vi "Main.vi"() -> ()   [LabVIEW 2020]
doc: "This template is for the Queued Message Handler design pattern.\n\nThe Event Handling Loop generates messages based on user interface actions.\n\nThe Message Handling Loop processes messages generated by the Event Handling Loop, or by other messages. The messages are string values, so new messages can be added easily to the Message Cases case structure in the Message Handling Loop. Each message cluster can also provide an optional value for Message Data, which is a variant that can be converted to whatever message-specific data is required."
uses:
  SubVi/TypeDef2ndLoop.ctl
  controls/UI Data.ctl
  <vilib>/Utility/miscctls.llb/LVForegroundBackgroundColorsTypeDef.ctl
  <vilib>/Utility/miscctls.llb/LVStringsAndValuesArrayTypeDef_U16.ctl
  <vilib>/Analysis/3filter.llb/Savitzky-Golay Filter (DBL).vi
  support/Message Queue/Enqueue Message (Single).vi
  <vilib>/Utility/file.llb/Write Delimited Spreadsheet (DBL).vi
  <vilib>/Utility/error.llb/Error Cluster From Error Code.vi
  <vilib>/ErrorRing/Error Ring.xnode
  <vilib>/Analysis/6fits.llb/Confidence Interval (Gauss).vi
  support/Message Queue/Message Queue.lvlib
  support/User Event - Stop/User Event - Stop.lvlib
  <instrlib>/Ocean Optics 2000 4000/Ocean Optics 2000 4000.lvlib
  <vilib>/Analysis/NI_AALBase.lvlib
  <vilib>/Analysis/NI_AALPro.lvlib
panel:
  out "PlotMouseFollow":string
  in  "Tab Control":enum32{"Analysis and Aquisition", "HR4000 "}(tab)
  in  "Grid on graph":bool
  in  "20(I)/10(P)":bool
  in  "Intensity/dB":bool
  in  "AutoScale":bool
  in  "Tab small":enum32{"Data Operations", "Linfit View"}(tab)
  in  "Save to file 3":bool
  in  "FIlterType":u16(ring) items=["Savitzky-Golay"]
  in  "FIlterorder":u16(ring) items=["1st order poly.", "2nd order poly.", "3rd order poly.", "4th order poly.", "5th order poly. ", "6th order poly."]
  in  "Filter":bool
  in  "Remove negative values":bool
  out "Data(X/Y)":cluster{dbl[], dbl[]}[](array[cluster])
  in  "Interpolate":bool
  in  "PlotChooser 2":u16(ring) items=["6,5cm60000"]
  in  "MathNumber":dbl
  in  "Math":bool
  in  "Tab Math":u16(ring) items=["Multiply", "Divide", "Add", "Decrement"]
  in  "Normalise":bool
  in  "Save to file":bool
  out "Max":dbl
  out "Min":dbl
  out "Attenuation[dB/cm]":dbl
  out "Linfit":cluster{"X":dbl[], "Best Linear Fit":dbl[]}[](graph)
  out "Intercept":dbl
  in  "Save session":bool
  out "FWHM":dbl
  in  "End":dbl min=0.0 max=2000.0
  in  "Start":dbl min=0.0 max=2000.0
  out "Attenuation[dB/cm]":dbl
  in  "Reference":dbl
  out "Reference name":string
  out "Attenuation[dB]":string
  out "Integral":string
  in  "PlotChooser":u16(ring) items=["6,5cm60000"]
  in  "DownloadData":bool
  out "Spectras-Analiza":cluster{dbl[], dbl[]}[](graph)
  in  "Delete series":bool
  in  "Data Display":dbl[][](array[numeric])
  out "Lenght[cm]":string
  in  "LinearFit":bool
  in  "Light mode":bool
  in  "Grid":bool
  in  "Intensity/dB":bool
  in  "Delete last":bool
  in  "PlotChooser 3":u16(ring) items=["Aquired"]
  in  "DarkSpectrum":bool
  in  "Save current spectrum":bool
  out "Spectras-Analiza 2":cluster{dbl[], dbl[]}[](graph)
  in  "VISA resource name":refnum<visa-resource-name>
  in  "Connect":bool
  in  "Disconnect":bool
  in  "Integration time [us]":i32=1 min=1 max=500000
  in  "Send data":bool
  out "Connection status":errorcluster
  in  "Choose folder":path
  in  "Save to file 2":bool
  in  "Aquire":bool
  in  "AutoScale":bool
  in  "AqvOverTime":bool
  in  "Exit":bool
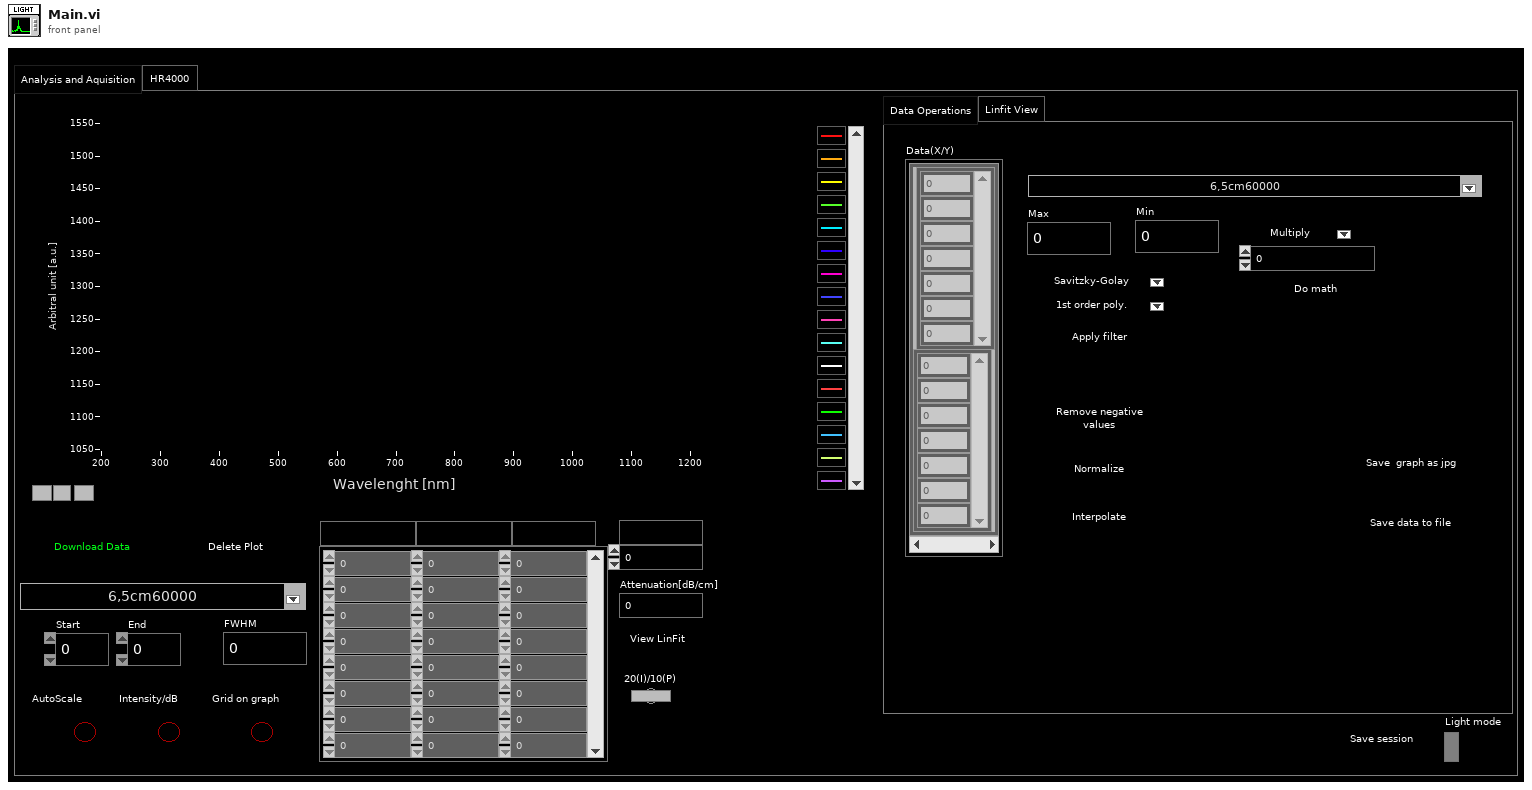
[diagram p1: front panel]
types:
  T1 = typedef "UI Data.ctl" = cluster{"Exit Button Ref":refnum<vi>, "Spectras-Analiza":cluster{dbl[], dbl[]}[], "PlotNumber":dbl, "DataDisplay":dbl[][], "VISA resource name":refnum<visa-resource-name>, "VISA error cluster":errorcluster, "Names of plots":cluster{"Plot.Plot Name":string, i32}[]}
  T2 = typedef "TypeDef2ndLoop.ctl" = cluster{"VISA resource name":refnum<visa-resource-name>, "VISA error cluster":errorcluster, "Spectras-Analiza":cluster{dbl[], dbl[]}[], "Spectral Waveform":cluster{dbl[], dbl[]}, "Spectrum by Pixel Number":dbl[], "Dark?":bool}
  T3 = typedef "Message Queue.lvlib/All Message Queues.ctl" = cluster{"1stloop":refnum<queue>, "2ndLoop":refnum<queue>}
  T4 = typedef "LVStringsAndValuesArrayTypeDef_U16.ctl" = cluster{"String":string, "Value":u16}[]
  T5 = enum8{"Enabled", "Disabled", "Disabled and Grayed Out"}
  T6 = cluster{"Wavelength (nm)":dbl[], "Spectrum by Pixel Number":dbl[]}
  T7 = typedef "LVForegroundBackgroundColorsTypeDef.ctl" = cluster{"Foreground Color":u32, "Background Color":u32}
  T8 = cluster{"name (change?)":string, "PlotNumber":dbl}[]
  T9 = typedef "LVPoint32TypeDef.ctl" = cluster{"Horizontal":i32, "Vertical":i32}
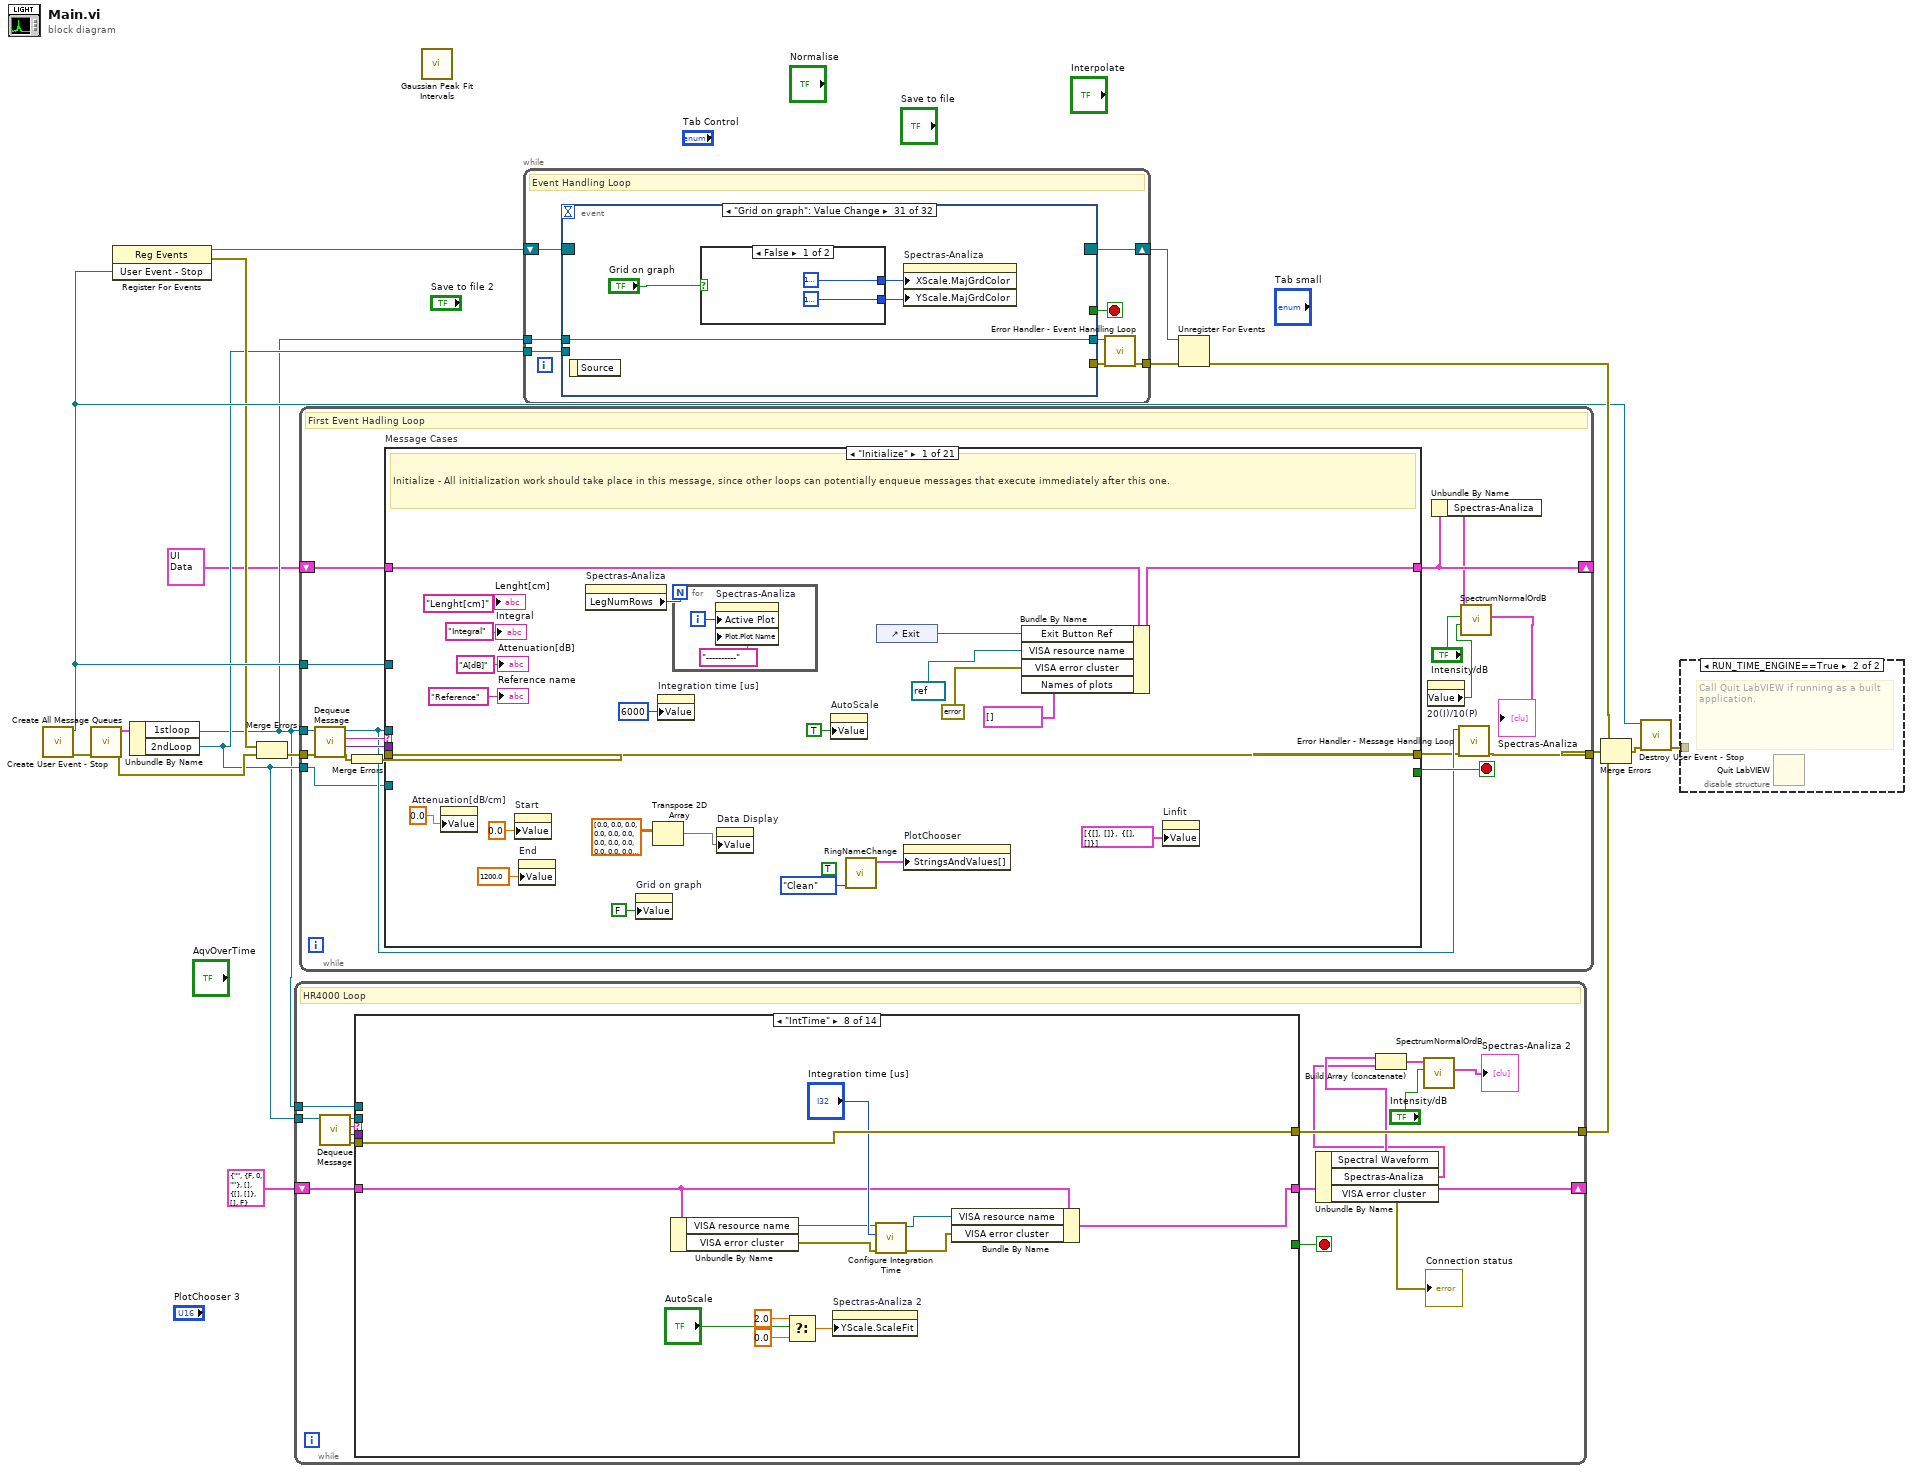
[diagram p0: block diagram]
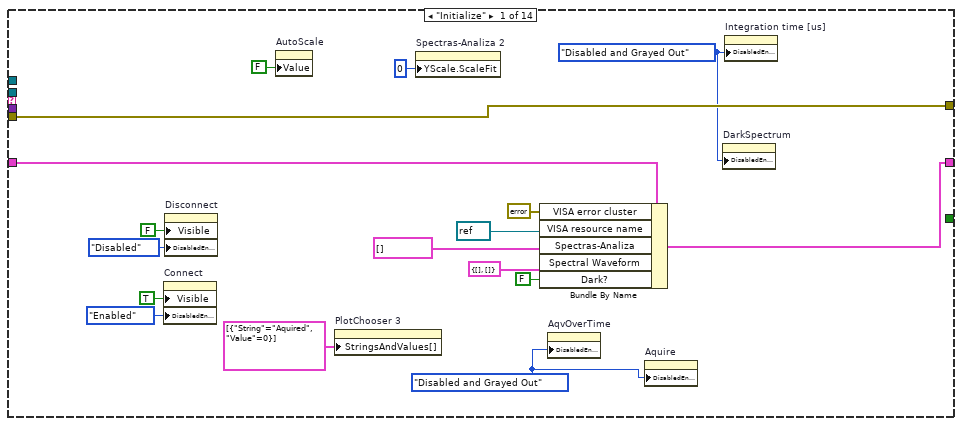
[diagram p2: hidden frame]
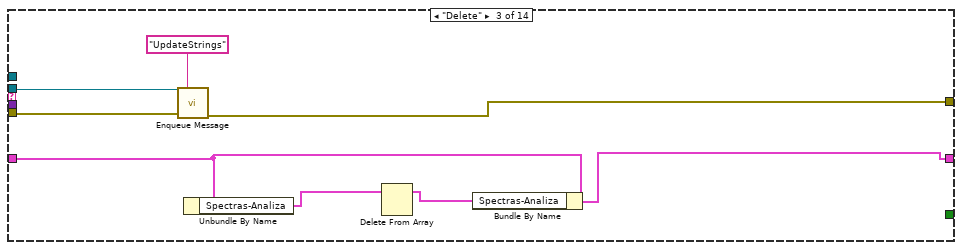
[diagram p4: hidden frame]
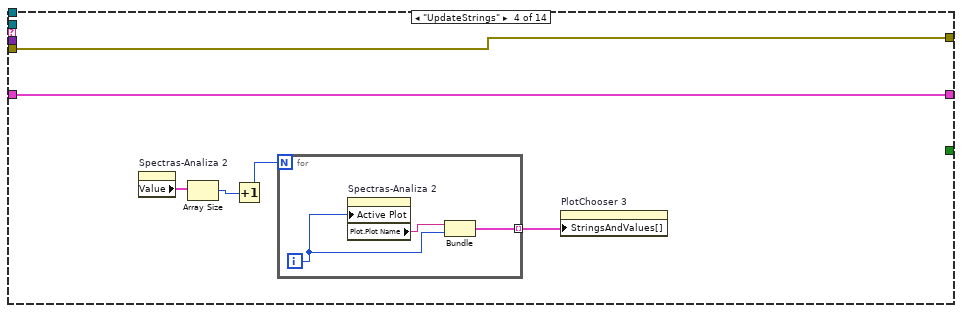
[diagram p5: hidden frame]
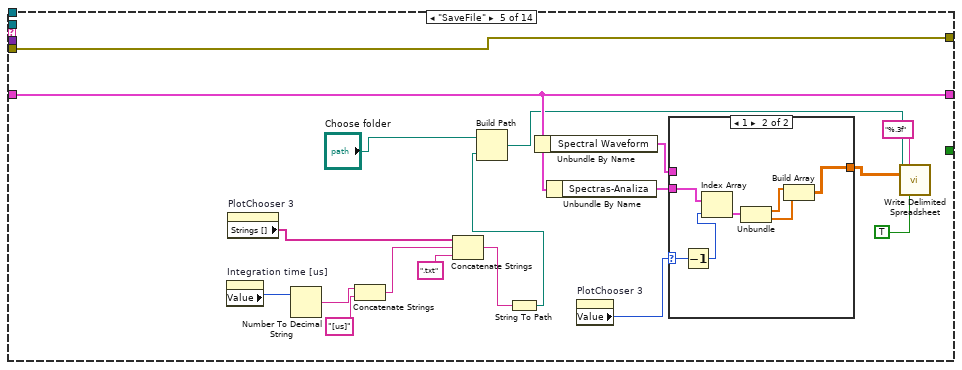
[diagram p6: hidden frame]
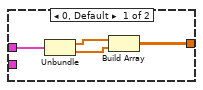
[diagram p7: hidden frame]
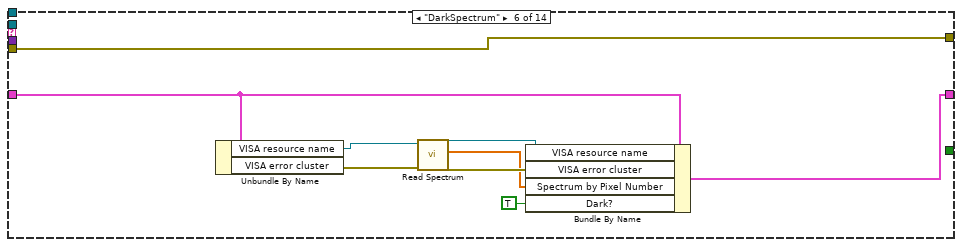
[diagram p8: hidden frame]
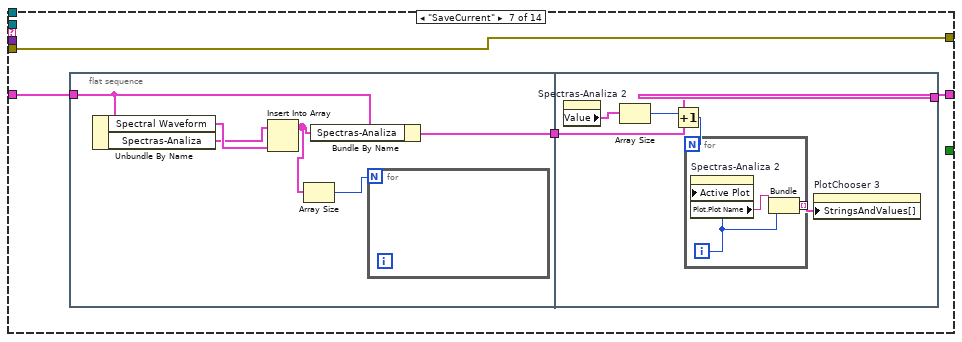
[diagram p9: hidden frame]
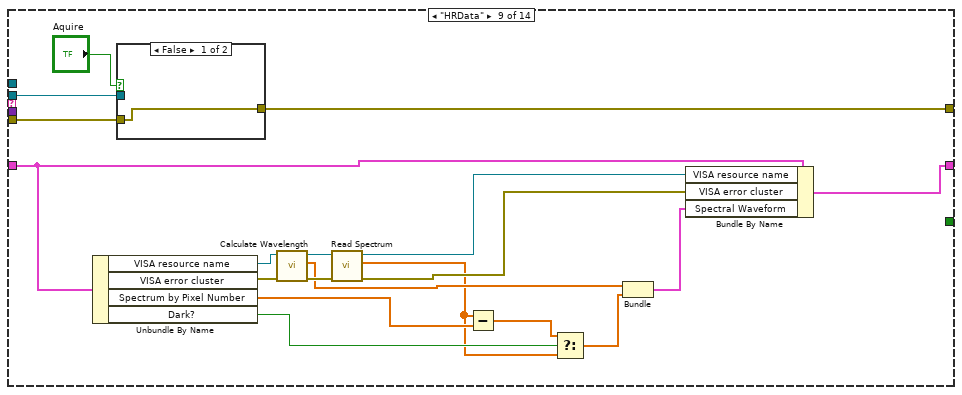
[diagram p10: hidden frame]
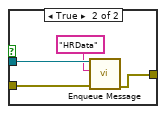
[diagram p11: hidden frame]
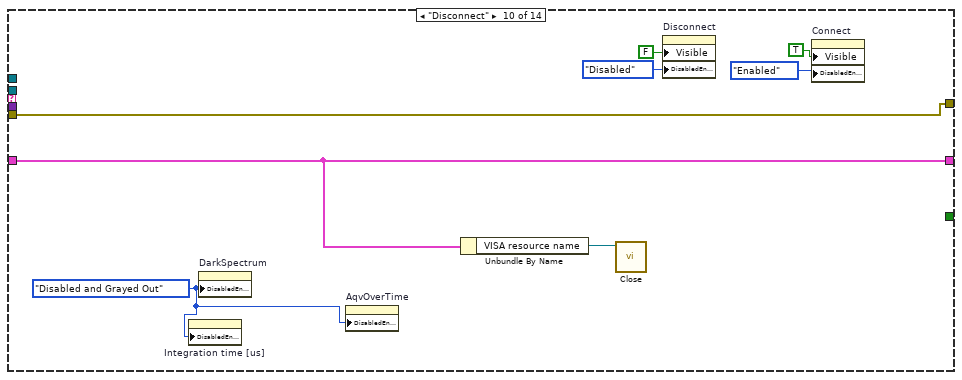
[diagram p12: hidden frame]
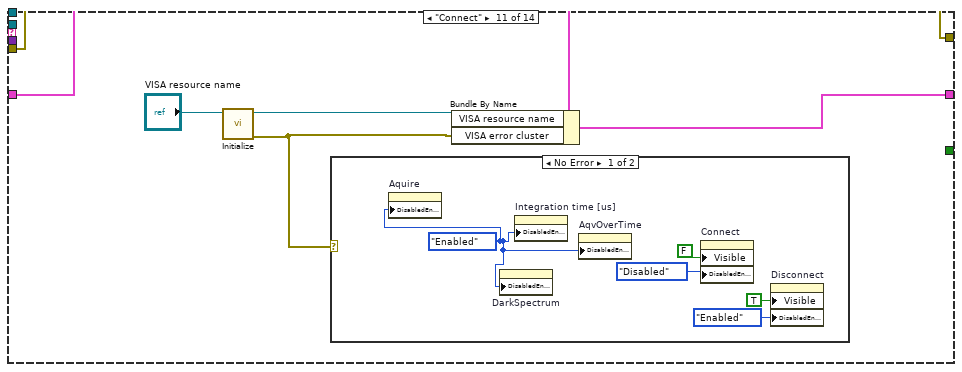
[diagram p13: hidden frame]
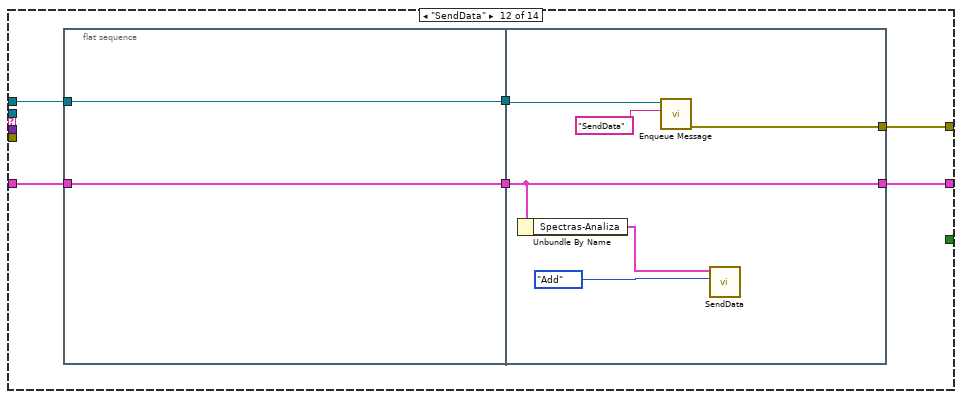
[diagram p15: hidden frame]
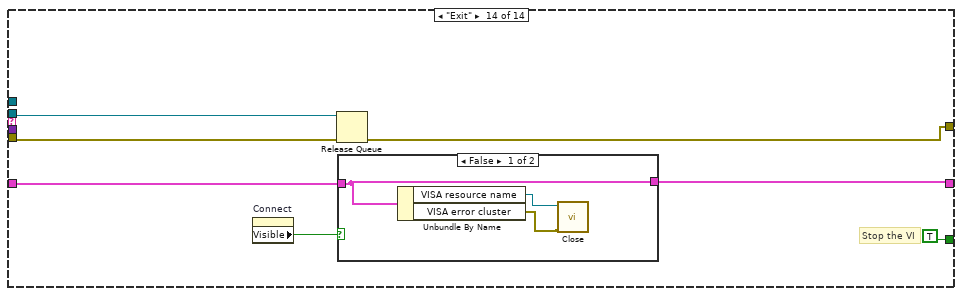
[diagram p17: hidden frame]
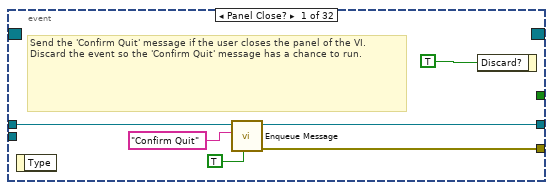
[diagram p20: hidden frame]
diagram:
  n1 = call "Create User Event - Stop.vi"() -> ("error out"=w15:errorcluster, "User Event - Stop"=w8:refnum<user-event>)  [unwired: 10 in]
  n2 = call "Create All Message Queues.vi"("error in (no error)"=w15) -> ("error out"=w18:errorcluster, "Message Queues out"=w17:T3)  [unwired: 9 in]
  n3 = register-events(w8) -> (reference out=w9:refnum<event-registration>, error out=w6:errorcluster)  [unwired: 2 in]
  n4 = Unbundle By Name(w17) -> ("1stloop"=w3:refnum<queue>, "2ndLoop"=w4:refnum<queue>)
  n5 = Merge Errors(w6, w18) -> (w7:errorcluster)
  n6 = while {
    tunnel: w4 -> [w33]
    tunnel: [w28] -> w5
    tunnel: w3 -> [w27]
    shift-right: [w25] -> _
    shift-left: T2 {"VISA resource name"="", "VISA error cluster"={"status"=FALSE, "code"=0, "source"=""}, "Spectras-Analiza"=[], "Spectral Waveform"={[], []}, "Spectrum by Pixel Number"=[], "Dark?"=FALSE} -> [w26]
    stop <- w34 stop-if-true
    # "HR4000 Loop"
    n7 = call "Dequeue Message.vi"("Message Queue"=w33) -> ("error out"=w30:errorcluster, "Message Data"=w31:variant, "Message"=w32:string, "dup Message Queue"=w29:refnum<queue>)  [unwired: 7 in]
    n8 = case shown="\"IntTime\"" w32 {
      tunnel: [_ _ _ _ _ _ _ _ _ _ _ _ _ TRUE] -> w34
      tunnel: w31 -> [_ _ _ _ _ _ _ _ _ _ _ _ _ _]
      tunnel: w30 -> [w51 w53 w56 w67 w88 w108 w112 w138 w155 w164 w172 _ w197 w202]
      tunnel: w29 -> [_ _ w57 _ _ _ _ _ w153 _ _ _ _ w203]
      tunnel: [w51 w53 w55 w67 w88 w108 w112 w138 w154 w164 w172 w185 w197 w198] -> w28
      tunnel: w27 -> [_ _ _ _ _ _ _ _ _ _ _ w187 _ _]
      tunnel: w26 -> [w49 w52 w60 w66 w77 w105 w111 w134 w157 w165 w176 w182 w196 w200]
      tunnel: [w50 w52 w58 w66 w77 w101 w110 w131 w156 w165 w175 w184 w196 w199] -> w25
      frame "Initialize" {
        w35 = T5."Disabled and Grayed Out" ("Disabled")
        w37 = T5."Disabled and Grayed Out" ("Disabled")
        n9 = property on="Connect" class="Bool"("Visible"=TRUE, "DisabledEnum"=T5."Enabled" ("Disabled")) -> ()  [unwired: 2 in, 2 out]
        n10 = property on="Disconnect" class="Bool"("Visible"=FALSE, "DisabledEnum"=T5."Disabled" ("Disabled")) -> ()  [unwired: 2 in, 2 out]
        n11 = property on="AutoScale" class="Bool (strict)"("Value"=FALSE ("AutoScale")) -> ()  [unwired: 2 in, 2 out]
        n12 = property on="PlotChooser 3" class="Ring (strict)"("StringsAndValues[]"=T4 [{"String"="Aquired", "Value"=0}] ("Strings And Values []")) -> ()  [unwired: 2 in, 2 out]
        n13 = property on="Spectras-Analiza 2" class="XYGraph (strict)"("YScale.ScaleFit"=u8 0 ("Y Scale.Scale Fit")) -> ()  [unwired: 2 in, 2 out]
        n14 = Bundle By Name(cluster=w49, "VISA error cluster"=errorcluster {"status"=FALSE, "code"=0, "source"=""}, "VISA resource name"=refnum<visa-resource-name> refnum, "Spectras-Analiza"=cluster{dbl[], dbl[]}[] [], "Spectral Waveform"=cluster{dbl[], dbl[]} {[], []}, "Dark?"=FALSE) -> (w50:T2)
        n15 = property on="AqvOverTime" class="Bool (strict)"("DisabledEnum"=w35) -> ()  [unwired: 2 in, 2 out]
        n16 = property on="Aquire" class="Bool (strict)"("DisabledEnum"=w35) -> ()  [unwired: 2 in, 2 out]
        n17 = property on="DarkSpectrum" class="Bool"("DisabledEnum"=w37) -> ()  [unwired: 2 in, 2 out]
        n18 = property on="Integration time [us]" class="DigNum (strict)"("DisabledEnum"=w37) -> ()  [unwired: 2 in, 2 out]
      }
      frame "---Copy This Case---" {
      }
      frame "Delete" {
        n19 = call-poly "Enqueue Message.vi"("error in (no error)"=w56, "Message"="UpdateStrings", "Message Queue"=w57) -> ("error out"=w55:errorcluster)  [unwired: 7 in, 1 out]
        n20 = Unbundle By Name(w60) -> ("Spectras-Analiza"=w61:cluster{dbl[], dbl[]}[])
        n21 = Delete From Array(array=w61) -> (array with subset deleted=w59:cluster{dbl[], dbl[]}[])  [unwired: 2 in, 1 out]
        n22 = Bundle By Name(cluster=w60, "Spectras-Analiza"=w59) -> (w58:T2)
      }
      frame "UpdateStrings" {
        n23 = property on="Spectras-Analiza 2" class="XYGraph (strict)"() -> ("Value"=w65:cluster{dbl[], dbl[]}[])  [unwired: 2 in, 2 out]
        n24 = Array Size(array=w65) -> (size(s)=w64:i32)
        n25 = Increment(x=w64) -> (x+1=w63:i32)
        n26 = for {
          N: w63 -> [_]
          tunnel: [w68] -> w62 mode=indexing
          i -> [w69]
          n27 = property on="Spectras-Analiza 2" class="XYGraph (strict)"("Active Plot"=w69) -> ("Plot.Plot Name"=w70:string)  [unwired: 2 in, 2 out]
          n28 = Bundle("Plot.Plot Name"=w70, w69) -> (w68:cluster{"Plot.Plot Name":string, i32})  [unwired: 1 in]
        }
        n29 = property on="PlotChooser 3" class="Ring (strict)"("StringsAndValues[]"=w62) -> ()  [unwired: 2 in, 2 out]
      }
      frame "SaveFile" {
        n30 = property on="Integration time [us]" class="DigNum (strict)"() -> ("Value"=w83:i32)  [unwired: 2 in, 2 out]
        n31 = property on="PlotChooser 3" class="Ring (strict)"() -> ("Strings []"=w85:string[])  [unwired: 2 in, 2 out]
        n32 = Number To Decimal String(number=w83) -> (decimal integer string=w82:string)  [unwired: 1 in]
        n33 = Concatenate Strings(w82, "[us]" ("string")) -> (w80:string)
        n34 = Concatenate Strings(w85, w80, ".txt" ("string")) -> (w86:string)
        n35 = String To Path(string=w86) -> (path=w79:path)
        n36 = Build Path(base path="Choose folder", name or relative path=w79) -> (appended path=w74:path)
        n37 = Unbundle By Name(w77) -> ("Spectral Waveform"=w76:cluster{dbl[], dbl[]})
        n38 = Unbundle By Name(w77) -> ("Spectras-Analiza"=w75:cluster{dbl[], dbl[]}[])
        n39 = property on="PlotChooser 3" class="Ring (strict)"() -> ("Value"=w78:u16)  [unwired: 2 in, 2 out]
        n40 = case shown="1" w78 {
          selector: w78 -> [_ w98]
          tunnel: w76 -> [w92 _]
          tunnel: [w89 w93] -> w71
          tunnel: w75 -> [_ w99]
          frame 0, Default {
            n41 = Unbundle(w92) -> (w91:dbl[], w90:dbl[])
            n42 = Build Array(w91, w90) -> (w89:dbl[][])
          }
          frame 1 {
            n43 = Decrement(x=w98) -> (x-1=w97:u16)
            n44 = Index Array(array=w99, index=w97) -> (element=w96:cluster{dbl[], dbl[]})
            n45 = Unbundle(w96) -> (w95:dbl[], w94:dbl[])
            n46 = Build Array(w95, w94) -> (w93:dbl[][])
          }
        }
        n47 = call-poly <vilib>:"Write Delimited Spreadsheet.vi"("file path (dialog if empty)"=w74, "format (%.3f)"="%.3f", "2D data"=w71, "transpose? (no:F)"=TRUE) -> ()  [unwired: 10 in, 2 out]
      }
      frame "DarkSpectrum" {
        n48 = Unbundle By Name(w105) -> ("VISA resource name"=w107:refnum<visa-resource-name>, "VISA error cluster"=w106:errorcluster)
        n49 = call <instrlib>:"Read Spectrum.vi"("error in (no error)"=w106, "VISA resource name"=w107) -> ("error out"=w103:errorcluster, "Spectrum by Pixel Number"=w102:dbl[], "VISA resource name out"=w104:refnum<visa-resource-name>)  [unwired: 6 in, 1 out]
        n50 = Bundle By Name(cluster=w105, "VISA resource name"=w104, "VISA error cluster"=w103, "Spectrum by Pixel Number"=w102, "Dark?"=TRUE) -> (w101:T2)
      }
      frame "SaveCurrent" {
        n51 = flat-sequence {
          tunnel: w111 -> [w116]
          tunnel: [w115] -> w109
          tunnel: [w123] -> w110
          tunnel: w109 -> [w123]
          frame #0 {
            n52 = Unbundle By Name(w116) -> ("Spectral Waveform"=w118:cluster{dbl[], dbl[]}, "Spectras-Analiza"=w117:cluster{dbl[], dbl[]}[])
            n53 = Insert Into Array(array=w117, new element=w118) -> (w114:cluster{dbl[], dbl[]}[])  [unwired: 1 in]
            n54 = Array Size(array=w114) -> (size(s)=w113:i32)
            n55 = Bundle By Name(cluster=w116, "Spectras-Analiza"=w114) -> (w115:T2)
            n56 = for {
              N: w113 -> [_]
            }
          }
          frame #1 {
            n57 = property on="Spectras-Analiza 2" class="XYGraph (strict)"() -> ("Value"=w122:cluster{dbl[], dbl[]}[])  [unwired: 2 in, 2 out]
            n58 = Array Size(array=w122) -> (size(s)=w121:i32)
            n59 = Increment(x=w121) -> (x+1=w120:i32)
            n60 = for {
              N: w120 -> [_]
              tunnel: [w124] -> w119 mode=indexing
              i -> [w125]
              n61 = property on="Spectras-Analiza 2" class="XYGraph (strict)"("Active Plot"=w125) -> ("Plot.Plot Name"=w126:string)  [unwired: 2 in, 2 out]
              n62 = Bundle("Plot.Plot Name"=w126, w125) -> (w124:cluster{"Plot.Plot Name":string, i32})  [unwired: 1 in]
            }
            n63 = property on="PlotChooser 3" class="Ring (strict)"("StringsAndValues[]"=w119) -> ()  [unwired: 2 in, 2 out]
          }
        }
      }
      frame "IntTime" {
        n64 = Unbundle By Name(w134) -> ("VISA resource name"=w136:refnum<visa-resource-name>, "VISA error cluster"=w135:errorcluster)
        n65 = Select(t=2.0, s="AutoScale", f=0.0) -> (s? t:f=w129:dbl)
        n66 = property on="Spectras-Analiza 2" class="XYGraph (strict)"("YScale.ScaleFit"=w129) -> ()  [unwired: 2 in, 2 out]
        n67 = call <instrlib>:"Configure Integration Time.vi"("error in (no error)"=w135, "Integration Time (6000)"="Integration time [us]", "VISA resource name"=w136) -> ("error out"=w132:errorcluster, "VISA resource name out"=w133:refnum<visa-resource-name>)  [unwired: 7 in]
        n68 = Bundle By Name(cluster=w134, "VISA resource name"=w133, "VISA error cluster"=w132) -> (w131:T2)
      }
      frame "HRData" {
        n69 = Unbundle By Name(w157) -> ("VISA resource name"=w150:refnum<visa-resource-name>, "VISA error cluster"=w149:errorcluster, "Spectrum by Pixel Number"=w143:dbl[], "Dark?"=w142:bool)
        n70 = case shown="False" "Aquire" {
          tunnel: w155 -> [w158 w162]
          tunnel: [w158 w161] -> w154
          tunnel: w153 -> [_ w160]
          frame False {
          }
          frame True {
            n71 = call-poly "Enqueue Message.vi"("error in (no error)"=w162, "Message"="HRData", "Message Queue"=w160) -> ("error out"=w161:errorcluster)  [unwired: 7 in, 1 out]
          }
        }
        n72 = call <instrlib>:"Calculate Wavelength.vi"("error in (no error)"=w149, "VISA resource name"=w150) -> ("error out"=w148:errorcluster, "Wavelength (nm)"=w145:dbl[], "VISA resource name out"=w151:refnum<visa-resource-name>)  [unwired: 1 in, 6 out]
        n73 = call <instrlib>:"Read Spectrum.vi"("error in (no error)"=w148, "VISA resource name"=w151) -> ("error out"=w146:errorcluster, "Spectrum by Pixel Number"=w140:dbl[], "VISA resource name out"=w147:refnum<visa-resource-name>)  [unwired: 6 in, 1 out]
        n74 = Subtract(x=w140, y=w143) -> (x-y=w141:dbl[])
        n75 = Select(t=w141, s=w142, f=w140) -> (s? t:f=w139:dbl[])
        n76 = Bundle("Wavelength (nm)"=w145, "Spectrum by Pixel Number"=w139) -> (w144:T6)  [unwired: 1 in]
        n77 = Bundle By Name(cluster=w157, "VISA resource name"=w147, "VISA error cluster"=w146, "Spectral Waveform"=w144) -> (w156:T2)
      }
      frame "Disconnect" {
        w163 = T5."Disabled and Grayed Out" ("Disabled")
        n78 = property on="Integration time [us]" class="DigNum (strict)"("DisabledEnum"=w163) -> ()  [unwired: 2 in, 2 out]
        n79 = property on="DarkSpectrum" class="Bool"("DisabledEnum"=w163) -> ()  [unwired: 2 in, 2 out]
        n80 = property on="AqvOverTime" class="Bool (strict)"("DisabledEnum"=w163) -> ()  [unwired: 2 in, 2 out]
        n81 = Unbundle By Name(w165) -> ("VISA resource name"=w170:refnum<visa-resource-name>)
        n82 = call <instrlib>:"Close.vi"("VISA resource name"=w170) -> ()  [unwired: 10 in, 1 out]
        n83 = property on="Disconnect" class="Bool"("Visible"=FALSE, "DisabledEnum"=T5."Disabled" ("Disabled")) -> ()  [unwired: 2 in, 2 out]
        n84 = property on="Connect" class="Bool"("Visible"=TRUE, "DisabledEnum"=T5."Enabled" ("Disabled")) -> ()  [unwired: 2 in, 2 out]
      }
      frame "Connect" {
        n85 = call <instrlib>:"Initialize.vi"("VISA resource name"="VISA resource name") -> ("error out"=w171:errorcluster, "VISA resource name out"=w173:refnum<visa-resource-name>)  [unwired: 9 in]
        n86 = case shown="No Error" w171 {
          frame No Error {
            w177 = T5."Enabled" ("Disabled")
            n87 = property on="Aquire" class="Bool (strict)"("DisabledEnum"=w177) -> ()  [unwired: 2 in, 2 out]
            n88 = property on="DarkSpectrum" class="Bool"("DisabledEnum"=w177) -> ()  [unwired: 2 in, 2 out]
            n89 = property on="Integration time [us]" class="DigNum (strict)"("DisabledEnum"=w177) -> ()  [unwired: 2 in, 2 out]
            n90 = property on="AqvOverTime" class="Bool (strict)"("DisabledEnum"=w177) -> ()  [unwired: 2 in, 2 out]
            n91 = property on="Connect" class="Bool"("Visible"=FALSE, "DisabledEnum"=T5."Disabled" ("Disabled")) -> ()  [unwired: 2 in, 2 out]
            n92 = property on="Disconnect" class="Bool"("Visible"=TRUE, "DisabledEnum"=T5."Enabled" ("Disabled")) -> ()  [unwired: 2 in, 2 out]
          }
          frame Error {
          }
        }
        n93 = Bundle By Name(cluster=w176, "VISA resource name"=w173, "VISA error cluster"=w171) -> (w175:T2)
      }
      frame "SendData" {
        n94 = flat-sequence {
          tunnel: w187 -> [w189]
          tunnel: [w189] -> w186
          tunnel: [w188] -> w183
          tunnel: w182 -> [w188]
          tunnel: w186 -> [w194]
          tunnel: [w193] -> w185
          tunnel: [w191] -> w184
          tunnel: w183 -> [w191]
          frame #0 {
          }
          frame #1 {
            n95 = Unbundle By Name(w191) -> ("Spectras-Analiza"=w190:cluster{dbl[], dbl[]}[])
            n96 = call-poly "Enqueue Message.vi"("Message"="SendData", "Message Queue"=w194) -> ("error out"=w193:errorcluster)  [unwired: 8 in, 1 out]
            n97 = call "SendData.vi"("Enum"=enum16{"Add", "Take"}."Add", "Spectras-Analiza"=w190) -> ()  [unwired: 9 in, 1 out]
          }
        }
      }
      frame Default {
      }
      frame "Exit" {
        # "Stop the VI"
        n98 = property on="Connect" class="Bool"() -> ("Visible"=w201:bool)  [unwired: 2 in, 2 out]
        n99 = Release Queue(queue=w203, error in (no error)=w202) -> (error out=w198:errorcluster)  [unwired: 1 in, 2 out]
        n100 = case shown="False" w201 {
          tunnel: [w205 w208] -> w199
          tunnel: w200 -> [w205 w208]
          frame False {
            n101 = Unbundle By Name(w205) -> ("VISA resource name"=w207:refnum<visa-resource-name>, "VISA error cluster"=w206:errorcluster)
            n102 = call <instrlib>:"Close.vi"("error in (no error)"=w206, "VISA resource name"=w207) -> ()  [unwired: 9 in, 1 out]
          }
          frame True {
          }
        }
      }
    }
    n103 = Unbundle By Name(w25) -> ("Spectral Waveform"=w24:cluster{dbl[], dbl[]}, "Spectras-Analiza"=w23:cluster{dbl[], dbl[]}[], "VISA error cluster"=→"Connection status":errorcluster)
    n104 = Build Array (concatenate)(w24, w23) -> (w21:cluster{dbl[], dbl[]}[])
    n105 = call "SpectrumNormalOrdB.vi"("Normal/dB"="Intensity/dB", "Spectras-Analiza"=w21) -> ("Spectras-Analiza"=→"Spectras-Analiza 2":cluster{dbl[], dbl[]}[])  [unwired: 9 in]
  }
  n106 = while {
    tunnel: w3 -> [w220]
    shift-right: [w210] -> _
    shift-left: T1 {"Exit Button Ref"=refnum, "Spectras-Analiza"=[], "PlotNumber"=0.0, "DataDisplay"=[[0.0, 0.0, 0.0, 0.0, 0.0, 0.0, 0.0, 0.0, 0.0, 0.0], [0.0, 0.0, 0.0, 0.0, 0.0, 0.0, 0.0, 0.0, 0.0, 0.0], [0.0, 0.0, 0.0, 0.0, 0.0, 0.0, 0.0, 0.0, 0.0, 0.0]], "VISA resource name"="", "VISA error cluster"={"status"=FALSE, "code"=0, "source"=""}, "Names of plots"=[]} ("Data Cluster") -> [w226]
    tunnel: w8 -> [w224]
    tunnel: w7 -> [w223]
    tunnel: [w218] -> w16
    tunnel: w4 -> [w214]
    stop <- w225 stop-if-true
    # "First Event Hadling Loop"
    n107 = call "Dequeue Message.vi"("error in (no error)"=w223, "Message Queue"=w220) -> ("error out"=w216:errorcluster, "Message Data"=w221:variant, "Message"=w222:string, "dup Message Queue"=w219:refnum<queue>)  [unwired: 6 in]
    n108 = Merge Errors(w216) -> (w215:errorcluster)
    n109 = case "Message Cases" shown="\"Initialize\"" w222 {
      selector: w222 -> [_ _ _ _ _ _ _ _ _ _ _ _ _ _ _ _ _ _ _ _ w648]
      tunnel: w219 -> [_ w254 _ w269 w280 w295 w364 w383 _ w405 _ _ w439 w486 w546 w577 w603 _ _ w647 _]
      tunnel: w215 -> [w247 w252 w260 w268 w282 _ w366 w384 w402 w406 w417 w426 w442 w497 w549 w576 w602 w622 w632 w635 _]
      tunnel: [w247 w256 w258 w278 w293 w300 w378 w392 w401 w411 w415 w425 w444 w487 w553 w578 w609 w621 w626 w644 w649] -> w217
      tunnel: w226 -> [w232 w257 w259 w271 w288 w298 w350 w391 w400 w403 w416 w423 w443 w493 w552 w573 w610 w620 w631 w633 w650]
      tunnel: [w249 w257 w259 w270 w283 w299 w343 w391 w400 w410 w416 w423 w438 w490 w551 w574 w610 w620 w631 w633 w650] -> w210
      tunnel: [_ _ _ _ _ _ _ _ _ _ _ _ _ _ _ _ _ _ _ TRUE _] -> w225
      tunnel: w221 -> [_ _ _ _ _ _ _ _ _ _ _ _ _ _ _ _ _ _ w630 w639 _]
      tunnel: w224 -> [_ _ _ _ _ _ _ _ _ _ _ _ _ _ _ _ _ _ _ w643 _]
      tunnel: w214 -> [_ _ _ _ _ _ _ _ _ _ _ _ _ _ _ _ _ _ _ w638 _]
      frame "Initialize" {
        (unwired) TRUE ("Data aquired?")
        # "Initialize - All initialization work should take place in this message, since other loops can potentially enqueue messages that execute immediately after this one."
        n110 = property on="Attenuation[dB/cm]" class="DigNum (strict)"("Value"=0.0 ("Attenuation[all]")) -> ()  [unwired: 2 in, 2 out]
        n111 = property on="Start" class="DigNum (strict)"("Value"=0.0 ("Start")) -> ()  [unwired: 2 in, 2 out]
        n112 = property on="End" class="DigNum (strict)"("Value"=1200.0 ("End")) -> ()  [unwired: 2 in, 2 out]
        n113 = property on="Spectras-Analiza" class="XYGraph (strict)"() -> ("LegNumRows"=w231:u32)  [unwired: 2 in, 2 out]
        n114 = property on="Grid on graph" class="Bool (strict)"("Value"=FALSE ("Grid on graph")) -> ()  [unwired: 2 in, 2 out]
        n115 = Transpose 2D Array(2D array=dbl[][] [[0.0, 0.0, 0.0, 0.0, 0.0, 0.0, 0.0, 0.0, 0.0, 0.0], [0.0, 0.0, 0.0, 0.0, 0.0, 0.0, 0.0, 0.0, 0.0, 0.0], [0.0, 0.0, 0.0, 0.0, 0.0, 0.0, 0.0, 0.0, 0.0, 0.0]] ("Array")) -> (transposed array=w239:dbl[][])
        n116 = property on="Integration time [us]" class="DigNum (strict)"("Value"=6000 ("Integration time")) -> ()  [unwired: 2 in, 2 out]
        n117 = for {
          N: w231 -> [_]
          i -> [w251]
          n118 = property on="Spectras-Analiza" class="XYGraph (strict)"("Active Plot"=w251, "Plot.Plot Name"="----------") -> ()  [unwired: 2 in, 2 out]
        }
        n119 = property on="Data Display" class="Arr (strict)"("Value"=w239) -> ()  [unwired: 2 in, 2 out]
        n120 = property on="AutoScale" class="Bool (strict)"("Value"=TRUE ("AutoScale")) -> ()  [unwired: 2 in, 2 out]
        n121 = call "RingNameChange.vi"("Enum"=enum16{"Add", "Delete", "Clean"}."Clean") -> ("Strings&Arrays"=w237:T8)  [unwired: 10 in]
        n122 = control-ref of="Exit"() -> (w248:refnum<vi>)
        n123 = property on="PlotChooser" class="Ring (strict)"("StringsAndValues[]"=w237) -> ()  [unwired: 2 in, 2 out]
        n124 = Bundle By Name(cluster=w232, "Exit Button Ref"=w248, "VISA resource name"=refnum<visa-resource-name> refnum, "VISA error cluster"=errorcluster {"status"=FALSE, "code"=0, "source"=""}, "Names of plots"=cluster{"Plot.Plot Name":string, i32}[] []) -> (w249:T1)
        n125 = property on="Linfit" class="XYGraph (strict)"("Value"=cluster{"X":dbl[], "Best Linear Fit":dbl[]}[] [{"X"=[], "Best Linear Fit"=[]}, {"X"=[], "Best Linear Fit"=[]}] ("Linfit")) -> ()  [unwired: 2 in, 2 out]
        "Integral" <- "Integral" ("Integral")
        "Lenght[cm]" <- "Lenght[cm]" ("Lenght[cm]")
        "Attenuation[dB]" <- "A[dB]" ("Attenuation[dB]")
        "Reference name" <- "Reference" ("Attenuation[dB] 2")
      }
      frame "Confirm Quit" {
        # "#CodeNeeded - If you want to provide an \"Are you sure\" dialog (or some other notification) before the application exits, place that code here. This message is typically sent from a Panel Close? event."
        # "Confirm Quit - Message that can confirm whether or not the user wants to exit the application."
        n126 = call-poly "Enqueue Message.vi"("error in (no error)"=w252, "Message"="Exit", "Message Queue"=w254) -> ("error out"=w255:errorcluster)  [unwired: 7 in, 1 out]
        n127 = Merge Errors(w255) -> (w256:errorcluster)
      }
      frame "---Copy This Frame---" {
        # "Duplicate this frame when creating new messages.  Change this comment in the duplicated frame to describe this message."
        n128 = Merge Errors(w260) -> (w258:errorcluster)
      }
      frame "Filter" {
        # "Duplicate this frame when creating new messages.  Change this comment in the duplicated frame to describe this message."
        n129 = call-poly "Enqueue Message.vi"("error in (no error)"=w268, "Message"="Integral", "Message Queue"=w269) -> ("error out"=w267:errorcluster)  [unwired: 7 in, 1 out]
        n130 = Unbundle By Name(w271) -> ("Spectras-Analiza"=w264:cluster{dbl[], dbl[]}[])
        n131 = property on="PlotChooser 2" class="Ring (strict)"() -> ("Value"=w272:u16)  [unwired: 2 in, 2 out]
        n132 = Increment(x="FIlterorder") -> (x+1=w261:u16)
        n133 = Index Array(array=w264, index=w272) -> (element=w276:cluster{dbl[], dbl[]})
        n134 = Unbundle(w276) -> (w274:dbl[], w275:dbl[])
        n135 = call-poly <vilib>:"Savitzky-Golay Filter.vi"("polynomial order"=w261, "side points"=6, "X"=w275) -> ("Filtered X"=w273:dbl[])  [unwired: 7 in, 1 out]
        n136 = Bundle(w274, "Filtered X"=w273) -> (w263:cluster{dbl[], "Filtered X":dbl[]})  [unwired: 1 in]
        n137 = Merge Errors(w267) -> (w278:errorcluster)
        n138 = Replace Array Subset(array=w264, new element=w263, index=w272) -> (w262:cluster{dbl[], dbl[]}[])
        n139 = Bundle By Name(cluster=w271, "Spectras-Analiza"=w262) -> (w270:T1)
      }
      frame "DoAbsVal" {
        # "Duplicate this frame when creating new messages.  Change this comment in the duplicated frame to describe this message."
        n140 = call-poly "Enqueue Message.vi"("error in (no error)"=w282, "Message"="Integral", "Message Queue"=w280) -> ("error out"=w281:errorcluster)  [unwired: 7 in, 1 out]
        n141 = Unbundle By Name(w288) -> ("Spectras-Analiza"=w287:cluster{dbl[], dbl[]}[])
        n142 = property on="PlotChooser 2" class="Ring (strict)"() -> ("Value"=w286:u16)  [unwired: 2 in, 2 out]
        n143 = Index Array(array=w287, index=w286) -> (element=w292:cluster{dbl[], dbl[]})
        n144 = Unbundle(w292) -> (w290:dbl[], w291:dbl[])
        n145 = Absolute Value(x=w291) -> (abs(x)=w289:dbl[])
        n146 = Bundle(w290, w289) -> (w285:cluster{dbl[], dbl[]})  [unwired: 1 in]
        n147 = Merge Errors(w281) -> (w293:errorcluster)
        n148 = Replace Array Subset(array=w287, new element=w285, index=w286) -> (w284:cluster{dbl[], dbl[]}[])
        n149 = Bundle By Name(cluster=w288, "Spectras-Analiza"=w284) -> (w283:T1)
      }
      frame "DownloadData" {
        # "Duplicate this frame when creating new messages.  Change this comment in the duplicated frame to describe this message."
        n150 = flat-sequence {
          tunnel: w298 -> [w306]
          tunnel: [w309] -> w297
          tunnel: w295 -> [w301]
          tunnel: [w301] -> w294
          tunnel: [w341] -> w299
          tunnel: w297 -> [w341]
          tunnel: [w339] -> w296
          tunnel: w294 -> [w338]
          frame #0 {
            n151 = call "DownloadDataNewWindow.vi"() -> ("Data aquired?"=w305:bool, "Yaxis"=w307:dbl[], "Xaxis"=w308:dbl[], "name (change?)"=w304:string, "Single FIle?"=w303:bool, "Multiple Data"=w302:cluster{dbl[], dbl[]}[])  [unwired: 6 in]
            n152 = case shown="True" w303 {
              tunnel: [w310 w328] -> w309
              tunnel: w308 -> [_ w325]
              tunnel: w307 -> [_ w324]
              tunnel: w306 -> [w311 w323]
              tunnel: w305 -> [_ w322]
              tunnel: w304 -> [_ w321]
              tunnel: w302 -> [w313 _]
              frame False {
                n153 = Unbundle By Name(w311) -> ("Spectras-Analiza"=w314:cluster{dbl[], dbl[]}[])
                n154 = Insert Into Array(array=w314, new element=w313) -> (w312:cluster{dbl[], dbl[]}[])  [unwired: 1 in]
                n155 = Bundle By Name(cluster=w311, "Spectras-Analiza"=w312) -> (w310:T1)
              }
              frame True {
                n156 = property on="Spectras-Analiza" class="XYGraph (strict)"() -> ("Value"=w318:cluster{dbl[], dbl[]}[])  [unwired: 2 in, 2 out]
                n157 = case shown="True" w322 {
                  tunnel: w321 -> [_ w337]
                  tunnel: w323 -> [w333 w336]
                  tunnel: [w332 w334] -> w320
                  frame False {
                    n158 = Unbundle By Name(w333) -> ("PlotNumber"=w332:dbl)
                  }
                  frame True {
                    n159 = Unbundle By Name(w336) -> ("PlotNumber"=w335:dbl)
                    n160 = property on="Spectras-Analiza" class="XYGraph (strict)"("Active Plot"=w335, "Plot.Plot Name"=w337) -> ()  [unwired: 2 in, 2 out]
                    n161 = Increment(x=w335) -> (x+1=w334:dbl)
                  }
                }
                n162 = Array Size(array=w318) -> (size(s)=w317:i32)
                n163 = Increment(x=w317) -> (x+1=w316:i32)
                n164 = for {
                  N: w316 -> [_]
                  tunnel: [w331] -> w315 mode=indexing
                  i -> [w329]
                  n165 = property on="Spectras-Analiza" class="XYGraph (strict)"("Active Plot"=w329) -> ("Plot.Plot Name"=w330:string)  [unwired: 2 in, 2 out]
                  n166 = Bundle("Plot.Plot Name"=w330, w329) -> (w331:cluster{"Plot.Plot Name":string, i32})  [unwired: 1 in]
                }
                n167 = Unbundle By Name(w323) -> ("Spectras-Analiza"=w327:cluster{dbl[], dbl[]}[])
                n168 = Bundle("Xaxis"=w325, "Yaxis"=w324) -> (w326:cluster{"Xaxis":dbl[], "Yaxis":dbl[]})  [unwired: 1 in]
                n169 = Insert Into Array(array=w327, new element=w326) -> (w319:cluster{dbl[], dbl[]}[])  [unwired: 1 in]
                n170 = property on="PlotChooser" class="Ring (strict)"("StringsAndValues[]"=w315) -> ()  [unwired: 2 in, 2 out]
                n171 = property on="PlotChooser 2" class="Ring (strict)"("StringsAndValues[]"=w315) -> ()  [unwired: 2 in, 2 out]
                n172 = Bundle By Name(cluster=w323, "Spectras-Analiza"=w319, "PlotNumber"=w320, "Names of plots"=w315) -> (w328:T1)
              }
            }
          }
          frame #1 {
            n173 = call-poly "Enqueue Message.vi"("Message"="Integral", "Message Queue"=w338) -> ("error out"=w339:errorcluster)  [unwired: 8 in, 1 out]
          }
        }
        n174 = Merge Errors(w296) -> (w300:errorcluster)
      }
      frame "Integral" {
        # "Duplicate this frame when creating new messages.  Change this comment in the duplicated frame to describe this message."
        n175 = Unbundle By Name(w350) -> ("Spectras-Analiza"=w349:cluster{dbl[], dbl[]}[])
        n176 = property on="PlotChooser 2" class="Ring (strict)"() -> ("Value"=w348:u16)  [unwired: 2 in, 2 out]
        n177 = call-poly "Enqueue Message.vi"("error in (no error)"=w366, "Message"="FWHM", "Message Queue"=w364) -> ("error out"=w365:errorcluster)  [unwired: 7 in, 1 out]
        n178 = property on="20(I)/10(P)" class="Bool (strict)"() -> ("Value"=w351:bool)  [unwired: 2 in, 2 out]
        n179 = Index Array(array=w349, index=w348) -> (element=w347:cluster{dbl[], dbl[]})
        n180 = Unbundle(w347) -> (w346:dbl[])  [unwired: 1 out]
        n181 = call "LinearFit.vi"("End"="End", "Start"="Start", "10/20"=w351, "Data Cluster"=w350) -> ("X"=w359:dbl[], "intercept"=→"Intercept":dbl, "Best Linear Fit"=w360:dbl[], "slope"=→"Attenuation[dB/cm]" →"Attenuation[dB/cm]":dbl, "Y"=w358:dbl[])  [unwired: 3 in]
        n182 = Array Max & Min(array=w346) -> (max value=→"Max":dbl, min value=→"Min":dbl)  [unwired: 2 out]
        n183 = Bundle("X"=w359, "Y"=w358) -> (w357:cluster{"X":dbl[], "Y":dbl[]})  [unwired: 1 in]
        n184 = Bundle("X"=w359, "Best Linear Fit"=w360) -> (w356:cluster{"X":dbl[], "Best Linear Fit":dbl[]})  [unwired: 1 in]
        n185 = Build Array(w357, w356) -> (→"Linfit":cluster{"X":dbl[], "Best Linear Fit":dbl[]}[])
        n186 = property on="20(I)/10(P)" class="Bool (strict)"() -> ("Value"=w352:bool)  [unwired: 2 in, 2 out]
        n187 = Equal?(x="Reference", y=0.0) -> (x = y?=w375:bool)
        n188 = call "DataDisplaySubVi.vi"("End"="End", "Start"="Start", "10/20"=w352, "Reference"="Reference", "Data Display"="Data Display", "Data Cluster"=w350) -> ("Data display(transposed)"=w377:dbl[][], "Data display"=w373:dbl[][])  [unwired: 4 in]
        n189 = Index Array(array=w373, index (row)=0) -> (element=w371:dbl[])  [unwired: 1 in]
        n190 = Merge Errors(w365) -> (w378:errorcluster)
        n191 = Index Array(array=w371, index=0) -> (element=w369:dbl)
        n192 = Bundle By Name(cluster=w350, "DataDisplay"=w373) -> (w343:T1)
        n193 = Select(t=w369, s=w375, f="Reference") -> (s? t:f=w368:dbl)
        n194 = property on="Data Display" class="Arr (strict)"("Value"=w377) -> ()  [unwired: 2 in, 2 out]
        n195 = property on="Reference" class="DigNum (strict)"("Value"=w368) -> ()  [unwired: 2 in, 2 out]
        n196 = Unbundle By Name(w343) -> ("Spectras-Analiza"=→"Data(X/Y)":cluster{dbl[], dbl[]}[])
      }
      frame "FWHM" {
        # "Duplicate this frame when creating new messages.  Change this comment in the duplicated frame to describe this message."
        n197 = call-poly "Enqueue Message.vi"("error in (no error)"=w384, "Message"="Start/End", "Message Queue"=w383) -> ("error out"=w382:errorcluster)  [unwired: 7 in, 1 out]
        n198 = Unbundle By Name(w391) -> ("Spectras-Analiza"=w390:cluster{dbl[], dbl[]}[])
        n199 = property on="PlotChooser" class="Ring (strict)"() -> ("Value"=w389:u16)  [unwired: 2 in, 2 out]
        n200 = Index Array(array=w390, index=w389) -> (element=w388:cluster{dbl[], dbl[]})
        n201 = Unbundle(w388) -> (w387:dbl[], w386:dbl[])
        n202 = property on="Start" class="DigNum (strict)"() -> ("Value"=w380:dbl)  [unwired: 2 in, 2 out]
        n203 = property on="End" class="DigNum (strict)"() -> ("Value"=w379:dbl)  [unwired: 2 in, 2 out]
        n204 = call "FWHM.vi"("End"=w379, "Start"=w380, "Yaxis"=w386, "Xaxis"=w387) -> ("FWHM"=→"FWHM":dbl)  [unwired: 7 in]
        n205 = Merge Errors(w382) -> (w392:errorcluster)
      }
      frame "LinearFit" {
        # "Duplicate this frame when creating new messages.  Change this comment in the duplicated frame to describe this message."
        n206 = property on="20(I)/10(P)" class="Bool (strict)"() -> ("Value"=w393:bool)  [unwired: 2 in, 2 out]
        n207 = property on="Start" class="DigNum (strict)"() -> ("Value"=w396:dbl)  [unwired: 2 in, 2 out]
        n208 = property on="End" class="DigNum (strict)"() -> ("Value"=w395:dbl)  [unwired: 2 in, 2 out]
        n209 = call "LinearFit.vi"("End"=w395, "Start"=w396, "10/20"=w393, "Data Cluster"=w400) -> ("X"=w398:dbl[], "Best Linear Fit"=w397:dbl[], "slope"=w399:dbl, "Y"=w394:dbl[])  [unwired: 3 in, 1 out]
        n210 = call "LinearFitPlot.vi"("Y"=w394, "Best Linear Fit"=w397, "X"=w398, "slope"=w399) -> ()  [unwired: 8 in]
        n211 = Merge Errors(w402) -> (w401:errorcluster)
      }
      frame "DataDisplay" {
        # "Duplicate this frame when creating new messages.  Change this comment in the duplicated frame to describe this message."
        n212 = call-poly "Enqueue Message.vi"("error in (no error)"=w406, "Message"="Integral", "Message Queue"=w405) -> ("error out"=w404:errorcluster)  [unwired: 7 in, 1 out]
        n213 = property on="Data Display" class="Arr (strict)"() -> ("Value"=w409:dbl[][])  [unwired: 2 in, 2 out]
        n214 = Transpose 2D Array(2D array=w409) -> (transposed array=w408:dbl[][])
        n215 = Bundle By Name(cluster=w403, "DataDisplay"=w408) -> (w410:T1)
        n216 = Merge Errors(w404) -> (w411:errorcluster)
      }
      frame "PlotNamesChange" {
        # "Duplicate this frame when creating new messages.  Change this comment in the duplicated frame to describe this message."
        n217 = property on="Spectras-Analiza" class="XYGraph (strict)"() -> ("Value"=w414:cluster{dbl[], dbl[]}[])  [unwired: 2 in, 2 out]
        n218 = Array Size(array=w414) -> (size(s)=w413:i32)
        n219 = for {
          N: w413 -> [_]
          tunnel: [w418] -> w412 mode=indexing
          i -> [w419]
          n220 = property on="Spectras-Analiza" class="XYGraph (strict)"("Active Plot"=w419) -> ("Plot.Plot Name"=w420:string)  [unwired: 2 in, 2 out]
          n221 = Bundle("Plot.Plot Name"=w420, w419) -> (w418:cluster{"Plot.Plot Name":string, i32})  [unwired: 1 in]
        }
        n222 = property on="PlotChooser 2" class="Ring (strict)"("StringsAndValues[]"=w412) -> ()  [unwired: 2 in, 2 out]
        n223 = property on="PlotChooser" class="Ring (strict)"("StringsAndValues[]"=w412) -> ()  [unwired: 2 in, 2 out]
        n224 = Merge Errors(w417) -> (w415:errorcluster)
      }
      frame "UpdateNames" {
        # "Duplicate this frame when creating new messages.  Change this comment in the duplicated frame to describe this message."
        n225 = property on="Spectras-Analiza" class="XYGraph (strict)"() -> ("Value"=w424:cluster{dbl[], dbl[]}[])  [unwired: 2 in, 2 out]
        n226 = Array Size(array=w424) -> (size(s)=w422:i32)
        n227 = property on="Spectras-Analiza" class="XYGraph (strict)" props=["Active Plot", "Plot", "Plot Name"]() -> ()  [unwired: 2 in, 4 out]
        n228 = Increment(x=w422) -> (x+1=w421:i32)
        n229 = for {
          N: w421 -> [_]
          tunnel: w423 -> [w431]
          i -> [w429]
          n230 = Unbundle By Name(w431) -> ("Names of plots"=w430:cluster{"Plot.Plot Name":string, i32}[])
          n231 = Index Array(array=w430, index=w429) -> (element=w428:cluster{"Plot.Plot Name":string, i32})
          n232 = Unbundle(w428) -> ("Plot.Plot Name"=w427:string)  [unwired: 1 out]
          n233 = property on="Spectras-Analiza" class="XYGraph (strict)"("Active Plot"=w429, "Plot.Plot Name"=w427) -> ()  [unwired: 2 in, 2 out]
        }
        n234 = Merge Errors(w426) -> (w425:errorcluster)
      }
      frame "DeletePlot" {
        # "Duplicate this frame when creating new messages.  Change this comment in the duplicated frame to describe this message."
        n235 = flat-sequence {
          tunnel: w443 -> [w458]
          tunnel: w442 -> [w462]
          tunnel: [w462] -> w441
          tunnel: [w461] -> w440
          tunnel: w439 -> [w461]
          tunnel: [w455] -> w437
          tunnel: [w451] -> w436
          tunnel: w441 -> [w467]
          tunnel: w440 -> [w468]
          tunnel: w437 -> [w470]
          tunnel: w436 -> [w465]
          tunnel: [w469] -> w435
          tunnel: [w468] -> w434
          tunnel: [w467] -> w433
          tunnel: [w484] -> w438
          tunnel: w435 -> [w484]
          tunnel: w434 -> [w482]
          tunnel: w433 -> [w479]
          tunnel: [w477] -> w432
          frame #0 {
            n236 = Unbundle By Name(w458) -> ("PlotNumber"=w459:dbl)
            n237 = property on="Spectras-Analiza" class="XYGraph (strict)"() -> ("Value"=w460:cluster{dbl[], dbl[]}[])  [unwired: 2 in, 2 out]
            n238 = Array Size(array=w460) -> (size(s)=w452:i32)
            n239 = for {
              N: w452 -> [_]
              tunnel: [w463] -> w454 mode=indexing
              i -> [w464]
              n240 = property on="Spectras-Analiza" class="XYGraph (strict)"("Active Plot"=w464) -> ("Plot.Plot Name"=w463:string)  [unwired: 2 in, 2 out]
            }
            n241 = Decrement(x=w459) -> (x-1=w448:dbl)
            n242 = Less Than 0?(x=w448) -> (x < 0?=w450:bool)
            n243 = Select(t=0.0, s=w450, f=w448) -> (s? t:f=w447:dbl)
            n244 = Bundle By Name(cluster=w458, "PlotNumber"=w447) -> (w456:T1)
            n245 = property on="PlotChooser" class="Ring (strict)"() -> ("Value"=w453:u16)  [unwired: 2 in, 2 out]
            n246 = Unbundle By Name(w456) -> ("Names of plots"=w457:cluster{"Plot.Plot Name":string, i32}[])
            n247 = Delete From Array(array=w454, index=w453) -> (array with subset deleted=w451:string[])  [unwired: 1 in, 1 out]
            n248 = Delete From Array(array=w457, index=w453) -> (array with subset deleted=w446:cluster{"Plot.Plot Name":string, i32}[])  [unwired: 1 in, 1 out]
            n249 = call "Names of plots.vi"("Names of plots"=w446) -> ("Names of plots"=w445:cluster{"Plot.Plot Name":string, i32}[])  [unwired: 10 in]
            n250 = property on="PlotChooser 2" class="Ring (strict)"("StringsAndValues[]"=w445) -> ()  [unwired: 2 in, 2 out]
            n251 = property on="PlotChooser" class="Ring (strict)"("StringsAndValues[]"=w445) -> ()  [unwired: 2 in, 2 out]
            n252 = Bundle By Name(cluster=w456, "Names of plots"=w445) -> (w455:T1)
          }
          frame #1 {
            n253 = Unbundle By Name(w470) -> ("Spectras-Analiza"=w471:cluster{dbl[], dbl[]}[])
            n254 = Array Size(array=w465) -> (size(s)=w466:i32)
            n255 = for {
              N: w466 -> [_]
              tunnel: w465 -> [w476]
              i -> [w475]
              n256 = Index Array(array=w476, index=w475) -> (element=w474:string)
              n257 = property on="Spectras-Analiza" class="XYGraph (strict)"("Active Plot"=w475, "Plot.Plot Name"=w474) -> ()  [unwired: 2 in, 2 out]
            }
            n258 = Delete From Array(array=w471, index="PlotChooser") -> (array with subset deleted=w472:cluster{dbl[], dbl[]}[])  [unwired: 1 in, 1 out]
            n259 = Bundle By Name(cluster=w470, "Spectras-Analiza"=w472) -> (w469:T1)
          }
          frame #2 {
            n260 = call-poly "Enqueue Message.vi"("error in (no error)"=w479, "Message"="UpdateNames", "Message Queue"=w482) -> ("error out"=w480:errorcluster, "dup Message Queue"=w481:refnum<queue>)  [unwired: 7 in]
            n261 = call-poly "Enqueue Message.vi"("error in (no error)"=w480, "Message"="Integral", "Message Queue"=w481) -> ("error out"=w477:errorcluster)  [unwired: 7 in, 1 out]
          }
        }
        n262 = Merge Errors(w432) -> (w444:errorcluster)
      }
      frame "Math" {
        # "Duplicate this frame when creating new messages.  Change this comment in the duplicated frame to describe this message."
        n263 = Unbundle By Name(w493) -> ("Spectras-Analiza"=w496:cluster{dbl[], dbl[]}[])
        n264 = Index Array(array=w496, index="PlotChooser 2") -> (element=w494:cluster{dbl[], dbl[]})
        n265 = case shown="1" "Tab Math" {
          tunnel: w494 -> [w503 w517 w530 w541]
          tunnel: [w504 w518 w523 w534] -> w490
          tunnel: w493 -> [w506 w520 w525 w536]
          tunnel: "MathNumber" -> [w502 w511 w531 w542]
          tunnel: "PlotChooser 2" -> [w507 w521 w532 w543]
          frame 0, Default {
            n266 = Unbundle By Name(w506) -> ("Spectras-Analiza"=w508:cluster{dbl[], dbl[]}[])
            n267 = Unbundle(w503) -> (w500:dbl[], w501:dbl[])
            n268 = Multiply(x=w501, y=w502) -> (x*y=w499:dbl[])
            n269 = Bundle(w500, w499) -> (w498:cluster{dbl[], dbl[]})  [unwired: 1 in]
            n270 = Replace Array Subset(array=w508, new element=w498, index=w507) -> (w505:cluster{dbl[], dbl[]}[])
            n271 = Bundle By Name(cluster=w506, "Spectras-Analiza"=w505) -> (w504:T1)
          }
          frame 1 {
            n272 = Unbundle By Name(w520) -> ("Spectras-Analiza"=w522:cluster{dbl[], dbl[]}[])
            n273 = Equal To 0?(x=w511) -> (x = 0?=w512:bool)
            n274 = Unbundle(w517) -> (w515:dbl[], w516:dbl[])
            n275 = Select(t=1.0, s=w512, f=w511) -> (s? t:f=w509:dbl)
            n276 = Divide(x=w516, y=w509) -> (x/y=w514:dbl[])
            n277 = Bundle(w515, w514) -> (w513:cluster{dbl[], dbl[]})  [unwired: 1 in]
            n278 = Replace Array Subset(array=w522, new element=w513, index=w521) -> (w519:cluster{dbl[], dbl[]}[])
            n279 = Bundle By Name(cluster=w520, "Spectras-Analiza"=w519) -> (w518:T1)
          }
          frame 2 {
            n280 = Unbundle By Name(w525) -> ("Spectras-Analiza"=w533:cluster{dbl[], dbl[]}[])
            n281 = Unbundle(w530) -> (w528:dbl[], w529:dbl[])
            n282 = Add(x=w529, y=w531) -> (x+y=w527:dbl[])
            n283 = Bundle(w528, w527) -> (w526:cluster{dbl[], dbl[]})  [unwired: 1 in]
            n284 = Replace Array Subset(array=w533, new element=w526, index=w532) -> (w524:cluster{dbl[], dbl[]}[])
            n285 = Bundle By Name(cluster=w525, "Spectras-Analiza"=w524) -> (w523:T1)
          }
          frame 3 {
            n286 = Unbundle By Name(w536) -> ("Spectras-Analiza"=w544:cluster{dbl[], dbl[]}[])
            n287 = Unbundle(w541) -> (w539:dbl[], w540:dbl[])
            n288 = Subtract(x=w540, y=w542) -> (x-y=w538:dbl[])
            n289 = Bundle(w539, w538) -> (w537:cluster{dbl[], dbl[]})  [unwired: 1 in]
            n290 = Replace Array Subset(array=w544, new element=w537, index=w543) -> (w535:cluster{dbl[], dbl[]}[])
            n291 = Bundle By Name(cluster=w536, "Spectras-Analiza"=w535) -> (w534:T1)
          }
        }
        n292 = Unbundle By Name(w490) -> ("Spectras-Analiza"=w489:cluster{dbl[], dbl[]}[])
        n293 = Merge Errors(w497) -> (w488:errorcluster)
        n294 = property on="Data(X/Y)" class="Arr (strict)"("Value"=w489) -> ()  [unwired: 2 in, 2 out]
        n295 = call-poly "Enqueue Message.vi"("error in (no error)"=w488, "Message"="Integral", "Message Queue"=w486) -> ("error out"=w487:errorcluster)  [unwired: 7 in, 1 out]
      }
      frame "SendData" {
        # "Duplicate this frame when creating new messages.  Change this comment in the duplicated frame to describe this message."
        n296 = flat-sequence {
          tunnel: w552 -> [w561]
          tunnel: w549 -> [w555]
          tunnel: [w560] -> w548
          tunnel: [w555] -> w547
          tunnel: w546 -> [w554]
          tunnel: [w554] -> w545
          tunnel: [w564] -> w550
          tunnel: [w566] -> w551
          tunnel: w548 -> [w566]
          tunnel: w547 -> [w565]
          tunnel: w545 -> [w563]
          frame #0 {
            n297 = Unbundle By Name(w561) -> ("Spectras-Analiza"=w559:cluster{dbl[], dbl[]}[])
            n298 = call "SendData.vi"("Enum"=enum16{"Add", "Take"}."Take") -> ("Spectras-Analiza 2"=w556:cluster{dbl[], dbl[]}[])  [unwired: 10 in]
            n299 = Insert Into Array(array=w559, new element=w556) -> (w558:cluster{dbl[], dbl[]}[])  [unwired: 1 in]
            n300 = Bundle By Name(cluster=w561, "Spectras-Analiza"=w558) -> (w560:T1)
          }
          frame #1 {
            n301 = call-poly "Enqueue Message.vi"("error in (no error)"=w565, "Message"="Integral", "Message Queue"=w563) -> ("error out"=w564:errorcluster)  [unwired: 7 in, 1 out]
          }
        }
        n302 = Merge Errors(w550) -> (w553:errorcluster)
      }
      frame "Start/End" {
        # "Duplicate this frame when creating new messages.  Change this comment in the duplicated frame to describe this message."
        n303 = flat-sequence {
          tunnel: w577 -> [w580]
          tunnel: [w580] -> w572
          tunnel: w576 -> [w581]
          tunnel: [w581] -> w570
          tunnel: [w579] -> w568
          tunnel: w573 -> [w579]
          tunnel: w572 -> [w594]
          tunnel: [w594] -> w571
          tunnel: w570 -> [w593]
          tunnel: [w593] -> w569
          tunnel: w568 -> [w592]
          tunnel: [w592] -> w567
          tunnel: w571 -> [w598]
          tunnel: w569 -> [w597]
          tunnel: [w596] -> w575
          tunnel: [w595] -> w574
          tunnel: w567 -> [w595]
          frame #0 {
            n304 = Unbundle By Name(w579) -> ()  [unwired: 1 out]
            n305 = property on="End" class="DigNum (strict)"() -> ("Value"=w583:dbl)  [unwired: 2 in, 2 out]
            n306 = property on="Start" class="DigNum (strict)"() -> ("Value"=w582:dbl)  [unwired: 2 in, 2 out]
            n307 = Greater?(x=w582, y=w583) -> (0:w584:bool)
            n308 = case shown="False" w584 {
              tunnel: w583 -> [w587 _]
              tunnel: w582 -> [w586 _]
              frame False {
                n309 = Less?(x=w587, y=w586) -> (x < y?=w585:bool)
                n310 = case shown="True" w585 {
                  frame False {
                  }
                  frame True {
                    n311 = property on="End" class="DigNum (strict)"() -> ("Value"=w589:dbl)  [unwired: 2 in, 2 out]
                    n312 = Increment(x=w589) -> (x+1=w588:dbl)
                    n313 = property on="Start" class="DigNum (strict)"("Value"=w588) -> ()  [unwired: 2 in, 2 out]
                  }
                }
              }
              frame True {
                n314 = property on="Start" class="DigNum (strict)"() -> ("Value"=w591:dbl)  [unwired: 2 in, 2 out]
                n315 = Increment(x=w591) -> (x+1=w590:dbl)
                n316 = property on="End" class="DigNum (strict)"("Value"=w590) -> ()  [unwired: 2 in, 2 out]
              }
            }
          }
          frame #1 {
          }
          frame #2 {
            n317 = call-poly "Enqueue Message.vi"("error in (no error)"=w597, "Message"="Integral", "Message Queue"=w598) -> ("error out"=w596:errorcluster)  [unwired: 7 in, 1 out]
          }
        }
        n318 = Merge Errors(w575) -> (w578:errorcluster)
      }
      frame "LightDarkMode" {
        # "Duplicate this frame when creating new messages.  Change this comment in the duplicated frame to describe this message."
        n319 = call-poly "Enqueue Message.vi"("error in (no error)"=w602, "Message"="Integral", "Message Queue"=w603) -> ("error out"=w601:errorcluster)  [unwired: 7 in, 1 out]
        n320 = case shown="True" "Light mode" {
          tunnel: [u32 16777225 ("X Scale.Name Label.Text Colors:Text Color") u32 0 ("X Scale.Name Label.Text Colors:Text Color")] -> w607
          tunnel: [u32 0 ("Frame Color") u32 16777215 ("Frame Color")] -> w606
          tunnel: [T7 {"Foreground Color"=0, "Background Color"=0} ("Plot Area:Colors") T7 {"Foreground Color"=16777225, "Background Color"=16777225} ("Plot Area:Colors")] -> w605
          tunnel: [u32 16777215 ("Frame Color") u32 0 ("Frame Color")] -> w600
          frame False {
          }
          frame True {
          }
        }
        n321 = property on="Spectras-Analiza" class="XYGraph (strict)"("Frame Color"=w606, "Plot Area Colors"=w605, "XScale.NameLbl.TextColor"=w607, "YScale.NameLbl.TextColor"=w607, "XScale.TickColor"=w600, "YScale.TickColor"=w600) -> ()  [unwired: 2 in, 2 out]
        n322 = Merge Errors(w601) -> (w609:errorcluster)
      }
      frame "Save session" {
        # "Duplicate this frame when creating new messages.  Change this comment in the duplicated frame to describe this message."
        n323 = property on="PlotChooser" class="Ring (strict)"() -> ("StringsAndValues[]"=w619:T4)  [unwired: 2 in, 2 out]
        n324 = while {
          shift-right: [w624] -> _
          shift-left: w620 -> [w624]
          shift-right: [w623] -> _
          shift-left: w619 -> [w623]
          stop <- TRUE stop-if-true
        }
        n325 = Merge Errors(w622) -> (w621:errorcluster)
      }
      frame "Error" {
        # "#CodeRecommended - If you ever change the name of this \"Error\" message, you'll need to update the name in the Check Loop Error.vi as well."
        # "#CodeRecommended - Consider creating a system for logging errors in some way. These errors are for notification purposes only. Handling of specific errors should be performed in the message frames that generated the error."
        # "Error - Display an error dialog. This message is sent by the \"Error Handler\" VIs at the end of other loops in this application."
        n326 = Variant To Data(error in=w632, type=errorcluster {"status"=FALSE, "code"=0, "source"=""} ("error constant"), Variant=w630) -> (data=w628:errorcluster, error out=w627:errorcluster)
        n327 = call <vilib>:"Simple Error Handler.vi"("error in (no error)"=w628) -> ()  [unwired: 4 in, 5 out]
        n328 = Merge Errors(w627) -> (w626:errorcluster)
      }
      frame "Exit" {
        # "Stop the VI"
        # "#CodeNeeded - Add any required cleanup code here. Note that if 'Exit' was called as a result of an error, an error dialog will be displayed. Add any custom error handling for an 'Exit' condition here as well."
        # "Exit - Exit the application."
        n329 = Variant To Data(type=errorcluster {"status"=FALSE, "code"=0, "source"=""} ("error constant"), Variant=w639) -> (data=w640:errorcluster)  [unwired: 1 in, 1 out]
        n330 = call <vilib>:"Simple Error Handler.vi"("error in (no error)"=w640) -> ()  [unwired: 4 in, 5 out]
        n331 = call "Fire User Event - Stop.vi"("User Event - Stop"=w643) -> ("error out"=w642:errorcluster)  [unwired: 10 in]
        n332 = Release Queue(queue=w647, error in (no error)=w635) -> (error out=w645:errorcluster)  [unwired: 1 in, 2 out]
        n333 = call-poly "Enqueue Message.vi"("Priority Message? (F)"=TRUE, "error in (no error)"=w635, "Message"="Exit", "Message Queue"=w638) -> ("error out"=w636:errorcluster)  [unwired: 6 in, 1 out]
        n334 = Merge Errors(w642, w645, w636) -> (w644:errorcluster)
      }
      frame Default {
        # "'Default' case only runs if there is a message that isn't defined in any of the other cases.  Output a programming error."
        n335 = xnode "Error Ring"("parameter 0"=w648) -> ("error out"=w649:errorcluster)
      }
    }
    n336 = property on="20(I)/10(P)" class="Bool (strict)"() -> ("Value"=w211:bool)  [unwired: 2 in, 2 out]
    n337 = Unbundle By Name(w210) -> ("Spectras-Analiza"=w209:cluster{dbl[], dbl[]}[])
    n338 = call "Error Handler - Message Handling Loop.vi"("error in (no error)"=w217, "Message Queue"=w219) -> ("dup error in"=w218:errorcluster)  [unwired: 8 in, 1 out]
    n339 = call "SpectrumNormalOrdB.vi"("20/10"=w211, "Normal/dB"="Intensity/dB", "Spectras-Analiza"=w209) -> ("Spectras-Analiza"=→"Spectras-Analiza":cluster{dbl[], dbl[]}[])  [unwired: 8 in]
  }
  n340 = call-poly <vilib>:"Gaussian Peak Fit Intervals.vi"() -> ()  [unwired: 10 in, 6 out]
  n341 = while {
    tunnel: w3 -> [w665]
    shift-right: [w663] -> w12
    shift-left: w9 -> [w664]
    tunnel: [w659] -> w10
    tunnel: w4 -> [w658]
    stop <- w661 stop-if-true
    # "Event Handling Loop"
    n342 = event shown="[30] \"Grid on graph\": Value Change" {
      selector: w664 -> [_ _ _ _ _ _ _ _ _ _ _ _ _ _ _ _ _ _ _ _ _ _ _ _ _ _ _ _ _ _ _ _]
      dyn-events: [_ _ _ _ _ _ _ _ _ _ _ _ _ _ _ _ _ _ _ _ _ _ _ _ _ _ _ _ _ _ _ _] -> w663
      timeout: _ -> [_ _ _ _ _ _ _ _ _ _ _ _ _ _ _ _ _ _ _ _ _ _ _ _ _ _ _ _ _ _ _ _]
      tunnel: [_ _ _ _ _ _ _ _ TRUE ("Discard?") _ _ _ _ _ _ _ _ _ _ _ _ _ _ _ _ _ _ _ _ _ _ _] -> w661
      tunnel: w665 -> [w670 w672 w677 w681 w684 _ _ w696 w699 w712 w716 w721 w727 w735 _ w744 _ w752 _ _ _ _ _ w777 _ w788 w792 w796 w800 w804 w808 w816]
      tunnel: [w669 _ w676 w679 w682 w687 w691 w694 _ _ w714 _ w725 w733 w738 w742 w747 w750 w754 w758 w762 w765 w770 _ w782 w786 w790 w793 w798 w802 _ _] -> w662
      tunnel: [w668 w672 w675 w680 w683 w688 w692 w695 w699 w712 w715 w721 w726 w734 w739 w743 w748 w751 w755 w759 w763 w766 w771 w777 w783 w787 w791 w795 w799 w803 w808 w816] -> w660
      tunnel: w658 -> [_ _ _ _ _ w686 w690 _ _ _ _ _ _ _ w740 _ w746 _ w756 w760 w764 w767 w772 _ w784 _ _ _ _ _ _ _]
      event Panel Close? {
        # "Send the 'Confirm Quit' message if the user closes the panel of the VI. Discard the event so the 'Confirm Quit' message has a chance to run."
        n343 = event-data() -> ()  [unwired: 1 in, 1 out]
        n344 = call-poly "Enqueue Message.vi"("Priority Message? (F)"=TRUE, "Message"="Confirm Quit", "Message Queue"=w670) -> ("error out"=w669:errorcluster, "dup Message Queue"=w668:refnum<queue>)  [unwired: 7 in]
        n345 = event-data("Discard?"=TRUE) -> ()  [unwired: 1 in, 1 out]
      }
      event Application Instance Close {
        # "#CodeRecommended - When a project closes, all VIs within that project are aborted and leave memory. However, any code placed in this event frame is guaranteed to run to completion, so add any cleanup code that absolutely must happen here."
        n346 = event-data() -> ()  [unwired: 1 in, 1 out]
      }
      event "Exit": Value Change {
        n347 = event-data() -> ()  [unwired: 1 in, 1 out]
        n348 = call-poly "Enqueue Message.vi"("Priority Message? (F)"=TRUE, "Message"="Exit", "Message Queue"=w677) -> ("error out"=w676:errorcluster, "dup Message Queue"=w675:refnum<queue>)  [unwired: 7 in]
      }
      event "DownloadData": Value Change {
        n349 = event-data() -> ()  [unwired: 1 in, 1 out]
        n350 = call-poly "Enqueue Message.vi"("Message"="DownloadData", "Message Queue"=w681) -> ("error out"=w679:errorcluster, "dup Message Queue"=w680:refnum<queue>)  [unwired: 8 in]
      }
      event "Light mode": Value Change {
        n351 = event-data() -> ()  [unwired: 1 in, 1 out]
        n352 = call-poly "Enqueue Message.vi"("Message"="LightDarkMode", "Message Queue"=w684) -> ("error out"=w682:errorcluster, "dup Message Queue"=w683:refnum<queue>)  [unwired: 8 in]
      }
      event "Connect": Value Change {
        n353 = event-data() -> ()  [unwired: 1 in, 1 out]
        n354 = call-poly "Enqueue Message.vi"("Message"="Connect", "Message Queue"=w686) -> ("error out"=w687:errorcluster, "dup Message Queue"=w688:refnum<queue>)  [unwired: 8 in]
      }
      event "Disconnect": Value Change {
        n355 = event-data() -> ()  [unwired: 1 in, 1 out]
        n356 = call-poly "Enqueue Message.vi"("Message"="Disconnect", "Message Queue"=w690) -> ("error out"=w691:errorcluster, "dup Message Queue"=w692:refnum<queue>)  [unwired: 8 in]
      }
      event "Start", "End": Value Change {
        n357 = event-data() -> ()  [unwired: 1 in, 1 out]
        n358 = call-poly "Enqueue Message.vi"("Message"="Start/End", "Message Queue"=w696) -> ("error out"=w694:errorcluster, "dup Message Queue"=w695:refnum<queue>)  [unwired: 8 in]
      }
      event User Event {
        # "The Message Handling Loop processed an \"Exit\" message, which fired this event to stop the Event Handling Loop."
        n359 = event-data() -> ()  [unwired: 1 in, 1 out]
      }
      event "Spectras-Analiza": Mouse Move {
        w708 = i16 2 ("precision (6)")
        n360 = event-data() -> ("Coords"=w701:T9)  [unwired: 1 in]
        n361 = invoke on="Spectras-Analiza" class="XYGraph (strict)" method="Map Coords To XY"("Coords"=w701) -> ("XY"=w711:cluster{"X":dbl, "Y":dbl})  [unwired: 6 in, 6 out]
        n362 = Unbundle(w711) -> ("X"=w710:dbl, "Y"=w709:dbl)
        n363 = invoke on="Spectras-Analiza" class="XYGraph (strict)" method="GetPlotAtPos"("InputPt"=w701) -> ("PlotNum"=w703:i32)  [unwired: 4 in, 4 out]
        n364 = Number To Fractional String(number=w709, precision (6)=w708) -> (F-format string=w706:string)  [unwired: 2 in]
        n365 = Number To Fractional String(number=w710, precision (6)=w708) -> (F-format string=w707:string)  [unwired: 2 in]
        n366 = Concatenate Strings(w707, "  " ("string"), w706) -> (w700:string)
        n367 = Not Equal?(x=-1, y=w703) -> (x != y?=w702:bool)
        n368 = property on="PlotMouseFollow" class="Str"("Visible"=w702, "Position"=w701, "Value"=w700) -> ()  [unwired: 2 in, 2 out]
      }
      event "Data Display", "Reference": Value Change {
        n369 = event-data() -> ()  [unwired: 1 in, 1 out]
        n370 = call-poly "Enqueue Message.vi"("Message"="DataDisplay", "Message Queue"=w716) -> ("error out"=w714:errorcluster, "dup Message Queue"=w715:refnum<queue>)  [unwired: 8 in]
      }
      event "AutoScale": Value Change {
        n371 = event-data() -> ()  [unwired: 1 in, 1 out]
        n372 = Select(t=2, s="AutoScale", f=0) -> (s? t:f=w717:i32)
        n373 = property on="Spectras-Analiza" class="XYGraph (strict)"("YScale.ScaleFit"=w717) -> ()  [unwired: 2 in, 2 out]
        n374 = property on="Spectras-Analiza" class="XYGraph (strict)"("XScale.ScaleFit"=w717) -> ()  [unwired: 2 in, 2 out]
      }
      event "Intensity/dB", "20(I)/10(P)": Value Change {
        n375 = event-data() -> ()  [unwired: 1 in, 1 out]
        n376 = property on="Intensity/dB" class="Bool (strict)"() -> ("Value"=w723:bool)  [unwired: 2 in, 2 out]
        n377 = case shown="True" w723 {
          tunnel: ["Arbitral unit [a.u.]" ("Y Scale.Name Label.Text") w731] -> w722
          frame False {
          }
          frame True {
            n378 = Select(t="10log(Unit)[dB]", s="20(I)/10(P)", f="20log(Unit)[dB]") -> (s? t:f=w731:string)
          }
        }
        n379 = call-poly "Enqueue Message.vi"("Message"="Integral", "Message Queue"=w727) -> ("error out"=w725:errorcluster, "dup Message Queue"=w726:refnum<queue>)  [unwired: 8 in]
        n380 = property on="Spectras-Analiza" class="XYGraph (strict)"("YScale.NameLbl.Text"=w722) -> ()  [unwired: 2 in, 2 out]
      }
      event "LinearFit": Value Change {
        n381 = event-data() -> ()  [unwired: 1 in, 1 out]
        n382 = call-poly "Enqueue Message.vi"("Message"="LinearFit", "Message Queue"=w735) -> ("error out"=w733:errorcluster, "dup Message Queue"=w734:refnum<queue>)  [unwired: 8 in]
      }
      event "Aquire": Value Change {
        n383 = event-data() -> ()  [unwired: 1 in, 1 out]
        n384 = call-poly "Enqueue Message.vi"("Message"="HRData", "Message Queue"=w740) -> ("error out"=w738:errorcluster, "dup Message Queue"=w739:refnum<queue>)  [unwired: 8 in]
      }
      event "Delete series": Value Change {
        n385 = event-data() -> ()  [unwired: 1 in, 1 out]
        n386 = call-poly "Enqueue Message.vi"("Message"="DeletePlot", "Message Queue"=w744) -> ("error out"=w742:errorcluster, "dup Message Queue"=w743:refnum<queue>)  [unwired: 8 in]
      }
      event "Send data": Value Change {
        n387 = event-data() -> ()  [unwired: 1 in, 1 out]
        n388 = call-poly "Enqueue Message.vi"("Message"="SendData", "Message Queue"=w746) -> ("error out"=w747:errorcluster, "dup Message Queue"=w748:refnum<queue>)  [unwired: 8 in]
      }
      event "Save session": Value Change {
        n389 = event-data() -> ()  [unwired: 1 in, 1 out]
        n390 = call-poly "Enqueue Message.vi"("Message"="Save session", "Message Queue"=w752) -> ("error out"=w750:errorcluster, "dup Message Queue"=w751:refnum<queue>)  [unwired: 8 in]
      }
      event "Integration time [us]": Value Change {
        n391 = event-data() -> ()  [unwired: 1 in, 1 out]
        n392 = call-poly "Enqueue Message.vi"("Message"="IntTime", "Message Queue"=w756) -> ("error out"=w754:errorcluster, "dup Message Queue"=w755:refnum<queue>)  [unwired: 8 in]
      }
      event "AutoScale": Value Change {
        n393 = event-data() -> ()  [unwired: 1 in, 1 out]
        n394 = call-poly "Enqueue Message.vi"("Message"="IntTime", "Message Queue"=w760) -> ("error out"=w758:errorcluster, "dup Message Queue"=w759:refnum<queue>)  [unwired: 8 in]
      }
      event "Save current spectrum": Value Change {
        n395 = event-data() -> ()  [unwired: 1 in, 1 out]
        n396 = call-poly "Enqueue Message.vi"("Message"="SaveCurrent", "Message Queue"=w764) -> ("error out"=w762:errorcluster, "dup Message Queue"=w763:refnum<queue>)  [unwired: 8 in]
      }
      event "DarkSpectrum": Value Change {
        n397 = event-data() -> ()  [unwired: 1 in, 1 out]
        n398 = call-poly "Enqueue Message.vi"("Message"="DarkSpectrum", "Message Queue"=w767) -> ("error out"=w765:errorcluster, "dup Message Queue"=w766:refnum<queue>)  [unwired: 8 in]
      }
      event "Save to file 2": Value Change {
        n399 = event-data() -> ()  [unwired: 1 in, 1 out]
        n400 = call-poly "Enqueue Message.vi"("Message"="SaveFile", "Message Queue"=w772) -> ("error out"=w770:errorcluster, "dup Message Queue"=w771:refnum<queue>)  [unwired: 8 in]
      }
      event "Spectras-Analiza 2": Plot Attribute Change {
        n401 = event-data() -> ()  [unwired: 1 in, 1 out]
        n402 = property on="Spectras-Analiza 2" class="XYGraph (strict)"() -> ("Value"=w776:cluster{dbl[], dbl[]}[])  [unwired: 2 in, 2 out]
        n403 = Array Size(array=w776) -> (size(s)=w775:i32)
        n404 = Increment(x=w775) -> (x+1=w774:i32)
        n405 = for {
          N: w774 -> [_]
          tunnel: [w780] -> w773 mode=indexing
          i -> [w778]
          n406 = property on="Spectras-Analiza 2" class="XYGraph (strict)"("Active Plot"=w778) -> ("Plot.Plot Name"=w779:string)  [unwired: 2 in, 2 out]
          n407 = Bundle("Plot.Plot Name"=w779, w778) -> (w780:cluster{"Plot.Plot Name":string, i32})  [unwired: 1 in]
        }
        n408 = property on="PlotChooser 3" class="Ring (strict)"("StringsAndValues[]"=w773) -> ()  [unwired: 2 in, 2 out]
      }
      event "Delete last": Value Change {
        n409 = event-data() -> ()  [unwired: 1 in, 1 out]
        n410 = call-poly "Enqueue Message.vi"("Message"="Delete", "Message Queue"=w784) -> ("error out"=w782:errorcluster, "dup Message Queue"=w783:refnum<queue>)  [unwired: 8 in]
      }
      event "Spectras-Analiza": Mouse Leave {
        n411 = event-data() -> ()  [unwired: 1 in, 4 out]
        n412 = call-poly "Enqueue Message.vi"("Message"="PlotNamesChange", "Message Queue"=w788) -> ("error out"=w786:errorcluster, "dup Message Queue"=w787:refnum<queue>)  [unwired: 8 in]
      }
      event "Math": Value Change {
        n413 = event-data() -> ()  [unwired: 1 in, 1 out]
        n414 = call-poly "Enqueue Message.vi"("Message"="Math", "Message Queue"=w792) -> ("error out"=w790:errorcluster, "dup Message Queue"=w791:refnum<queue>)  [unwired: 8 in]
      }
      event "PlotChooser 2": Value Change {
        n415 = event-data() -> ()  [unwired: 1 in, 1 out]
        n416 = call-poly "Enqueue Message.vi"("Message"="Integral", "Message Queue"=w796) -> ("error out"=w793:errorcluster, "dup Message Queue"=w795:refnum<queue>)  [unwired: 8 in]
      }
      event "Remove negative values": Value Change {
        n417 = event-data() -> ()  [unwired: 1 in, 1 out]
        n418 = call-poly "Enqueue Message.vi"("Message"="DoAbsVal", "Message Queue"=w800) -> ("error out"=w798:errorcluster, "dup Message Queue"=w799:refnum<queue>)  [unwired: 8 in]
      }
      event "Filter": Value Change {
        n419 = event-data() -> ()  [unwired: 1 in, 1 out]
        n420 = call-poly "Enqueue Message.vi"("Message"="Filter", "Message Queue"=w804) -> ("error out"=w802:errorcluster, "dup Message Queue"=w803:refnum<queue>)  [unwired: 8 in]
      }
      event "Grid on graph": Value Change {
        n421 = event-data() -> ()  [unwired: 1 in, 1 out]
        n422 = case shown="False" "Grid on graph" {
          tunnel: [u32 16777216 ("X Scale.Grid Colors:Major Color") u32 16777225 ("X Scale.Grid Colors:Major Color")] -> w806
          tunnel: [u32 16777216 ("Y Scale.Grid Colors:Major Color") u32 16777225 ("Y Scale.Grid Colors:Major Color")] -> w805
          frame False {
          }
          frame True {
          }
        }
        n423 = property on="Spectras-Analiza" class="XYGraph (strict)"("XScale.MajGrdColor"=w806, "YScale.MajGrdColor"=w805) -> ()  [unwired: 2 in, 2 out]
      }
      event "Grid": Value Change {
        n424 = event-data() -> ()  [unwired: 1 in, 1 out]
        n425 = case shown="True" "Grid" {
          tunnel: [u32 16777216 ("X Scale.Grid Colors:Major Color") u32 16777225 ("X Scale.Grid Colors:Major Color")] -> w814
          tunnel: [u32 16777216 ("Y Scale.Grid Colors:Major Color") u32 16777225 ("Y Scale.Grid Colors:Major Color")] -> w813
          frame False {
          }
          frame True {
          }
        }
        n426 = property on="Spectras-Analiza 2" class="XYGraph (strict)"("XScale.MajGrdColor"=w814, "YScale.MajGrdColor"=w813) -> ()  [unwired: 2 in, 2 out]
      }
    }
    n427 = call "Error Handler - Event Handling Loop.vi"("error in (no error)"=w662, "Message Queue"=w660) -> ("dup error in"=w659:errorcluster)  [unwired: 8 in, 1 out]
  }
  n428 = Unregister For Events(event registration refnum=w12, error in=w10) -> (error out=w13:errorcluster)
  n429 = Merge Errors(w13, w16, w5) -> (w14:errorcluster)
  n430 = call "Destroy User Event - Stop.vi"("error in (no error)"=w14, "User Event - Stop"=w8) -> ("error out"=w11:errorcluster)  [unwired: 9 in]
  n431 = disable-structure shown="RUN_TIME_ENGINE==True" {
    disable-tunnel: w11 -> [_ _]
    frame condition #0 (active) {
    }
    frame condition #1 {
      # "Call Quit LabVIEW if running as a built application."
      n432 = Quit LabVIEW() -> ()  [unwired: 1 in]
    }
  }
